vi "Main.vi"() -> ()   [LabVIEW 2016]
uses:
  <vilib>/picture/picture.llb/imagedata.ctl
panel:
  in  "Path 2":path
  in  "image data 2":T1 caption="图像数据"
  in  "Rectangle 2":T2
  out "Picture 2":picture
  in  "pConvertInfo In 4":T3
  in  "pConvertInfo In 3":T3
  out "frameHandle 2":i64
  out "Acquired Frames/s 2":dbl
  out "ResumeFlag 2":bool
  out "hDev 2":i64
  out "hIFDev 2":i64
  in  "ExposureAuto 2":i32(ring)
  in  "DeviceScanType 2":i32(ring) items=["Areascan", "Linescan"]
  out "InterfaceOpened 2":bool
  in  "Height 2":i32
  in  "Width 2":i32
  in  "PixelFormat 2":i32(ring)
  in  "GainRaw 2":dbl
  in  "ExposureTime 2":dbl
  out "IsGrabbing 2":bool
  out "TrigModeOn 2":bool
  in  "DeviceOpened 2":bool
  in  "DeviceList 2":i64(ring)
  out "ResumeFlag":bool
  in  "Path":path
  in  "SavePic":bool
  in  "pConvertInfo In 2":T3
  out "frameHandle":i64
  in  "DeviceInterfaceType":u16(ring) items=["GigE", "U3v", "CameraLink", "CXP"]
  in  "ExposureAuto":i32(ring)
  out "QuitFlag":bool
  in  "pConvertInfo In":T3
  in  "image data":T1 caption="图像数据"
  in  "Rectangle":T2
  in  "DeviceScanType":i32(ring) items=["Areascan", "Linescan"]
  out "InterfaceOpened":bool
  out "hDev":i64
  out "nInterfaceNum":u32
  out "hIFDev":i64
  out "interfaceKeyList":string[](array[string])
  out "HasInterface":bool
  out "Picture":picture
  out "Acquired Frames/s":dbl
  in  "TriggerSource":i32(ring)
  in  "ExecuteSoftTrig":bool
  in  "CloseTrig":bool
  in  "OpenTrig":bool
  in  "Stop":bool
  in  "Play":bool
  in  "Quit":bool
  in  "Height":i32
  in  "Width":i32
  in  "PixelFormat":i32(ring)
  in  "GainRaw":dbl
  in  "ExposureTime":dbl
  out "IsGrabbing":bool
  out "TrigModeOn":bool
  out "error out":errorcluster
  in  "error in":errorcluster
  in  "Close":bool
  in  "Open":bool
  out "HasDevices":bool
  in  "DeviceOpened":bool
  in  "DeviceList":i64(ring)
  in  "Discovery":bool
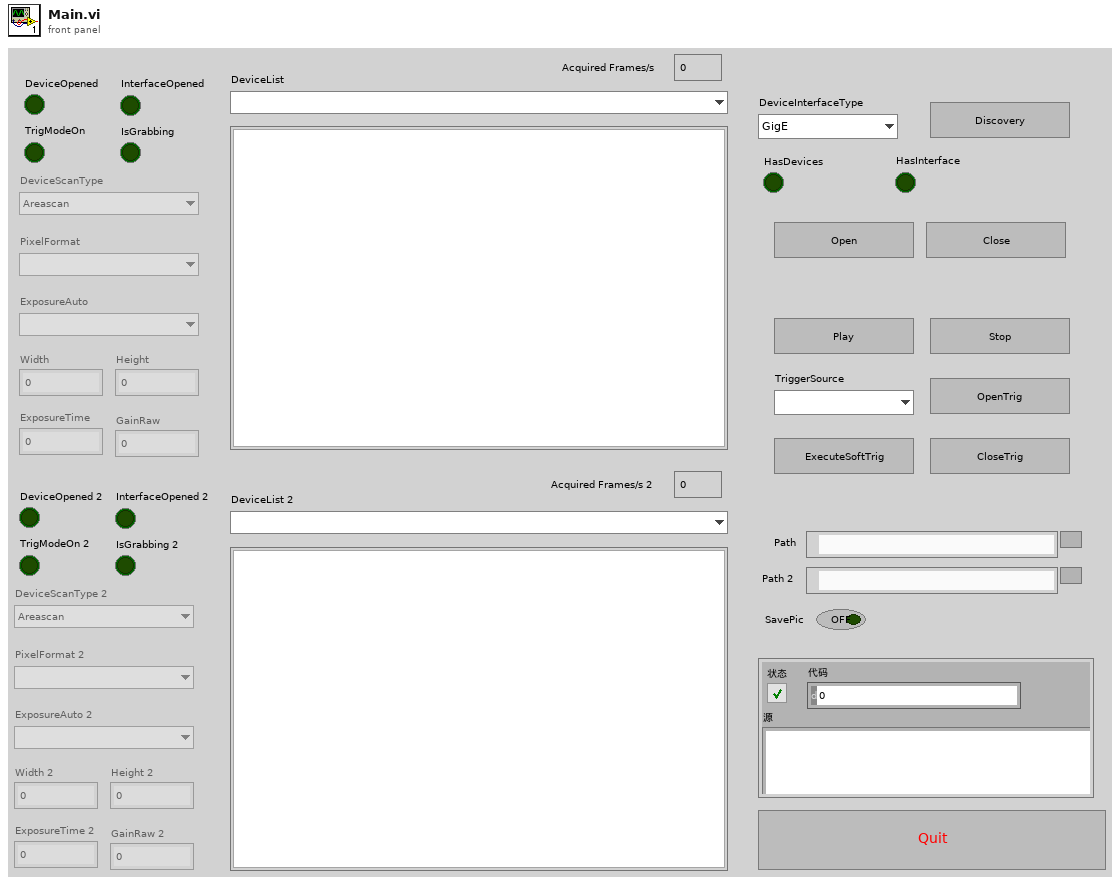
[diagram p1: front panel]
types:
  T1 = typedef "imagedata.ctl" = cluster{"image type":i32, "image depth":i32, "image":u8[], "mask":u8[], "colors":u32[], "Rectangle":cluster{"left":i16, "top":i16, "right":i16, "bottom":i16}}
  T2 = cluster{"left":i16, "top":i16, "right":i16, "bottom":i16}
  T3 = cluster{"nWidth":u32, "nHeight":u32, "enSrcPixelType":u32, "nSrcDataLen":u32, "nPaddingX":u32, "nPaddingY":u32, "eBayerDemosaic":u32, "eDstPixelFormat":u32, "nDstBufSize":u32, "nDstDataLen":u32, "nReserved0":u32, "nReserved1":u32, "nReserved2":u32, "nReserved3":u32, "nReserved4":u32, "nReserved5":u32, "nReserved6":u32, "nReserved7":u32}
  T4 = cluster{"blockId":u64, "status":u32, "width":u32, "height":u32, "size":u32, "pixelFormat":u32, "timeStamp":u64, "chunkCount":u32, "paddingX":u32, "paddingY":u32, "recvFrameTime":u32}
  T5 = cluster{"blockId":u64, "status":u32, "width":u32, "height":u32, "size":u32, "pixelFormat":i32, "timeStamp":u64, "chunkCount":u32, "paddingX":u32, "paddingY":u32, "recvFrameTime":u32}
  T6 = enum8{"Enabled", "Disabled", "Disabled and Grayed Out"}
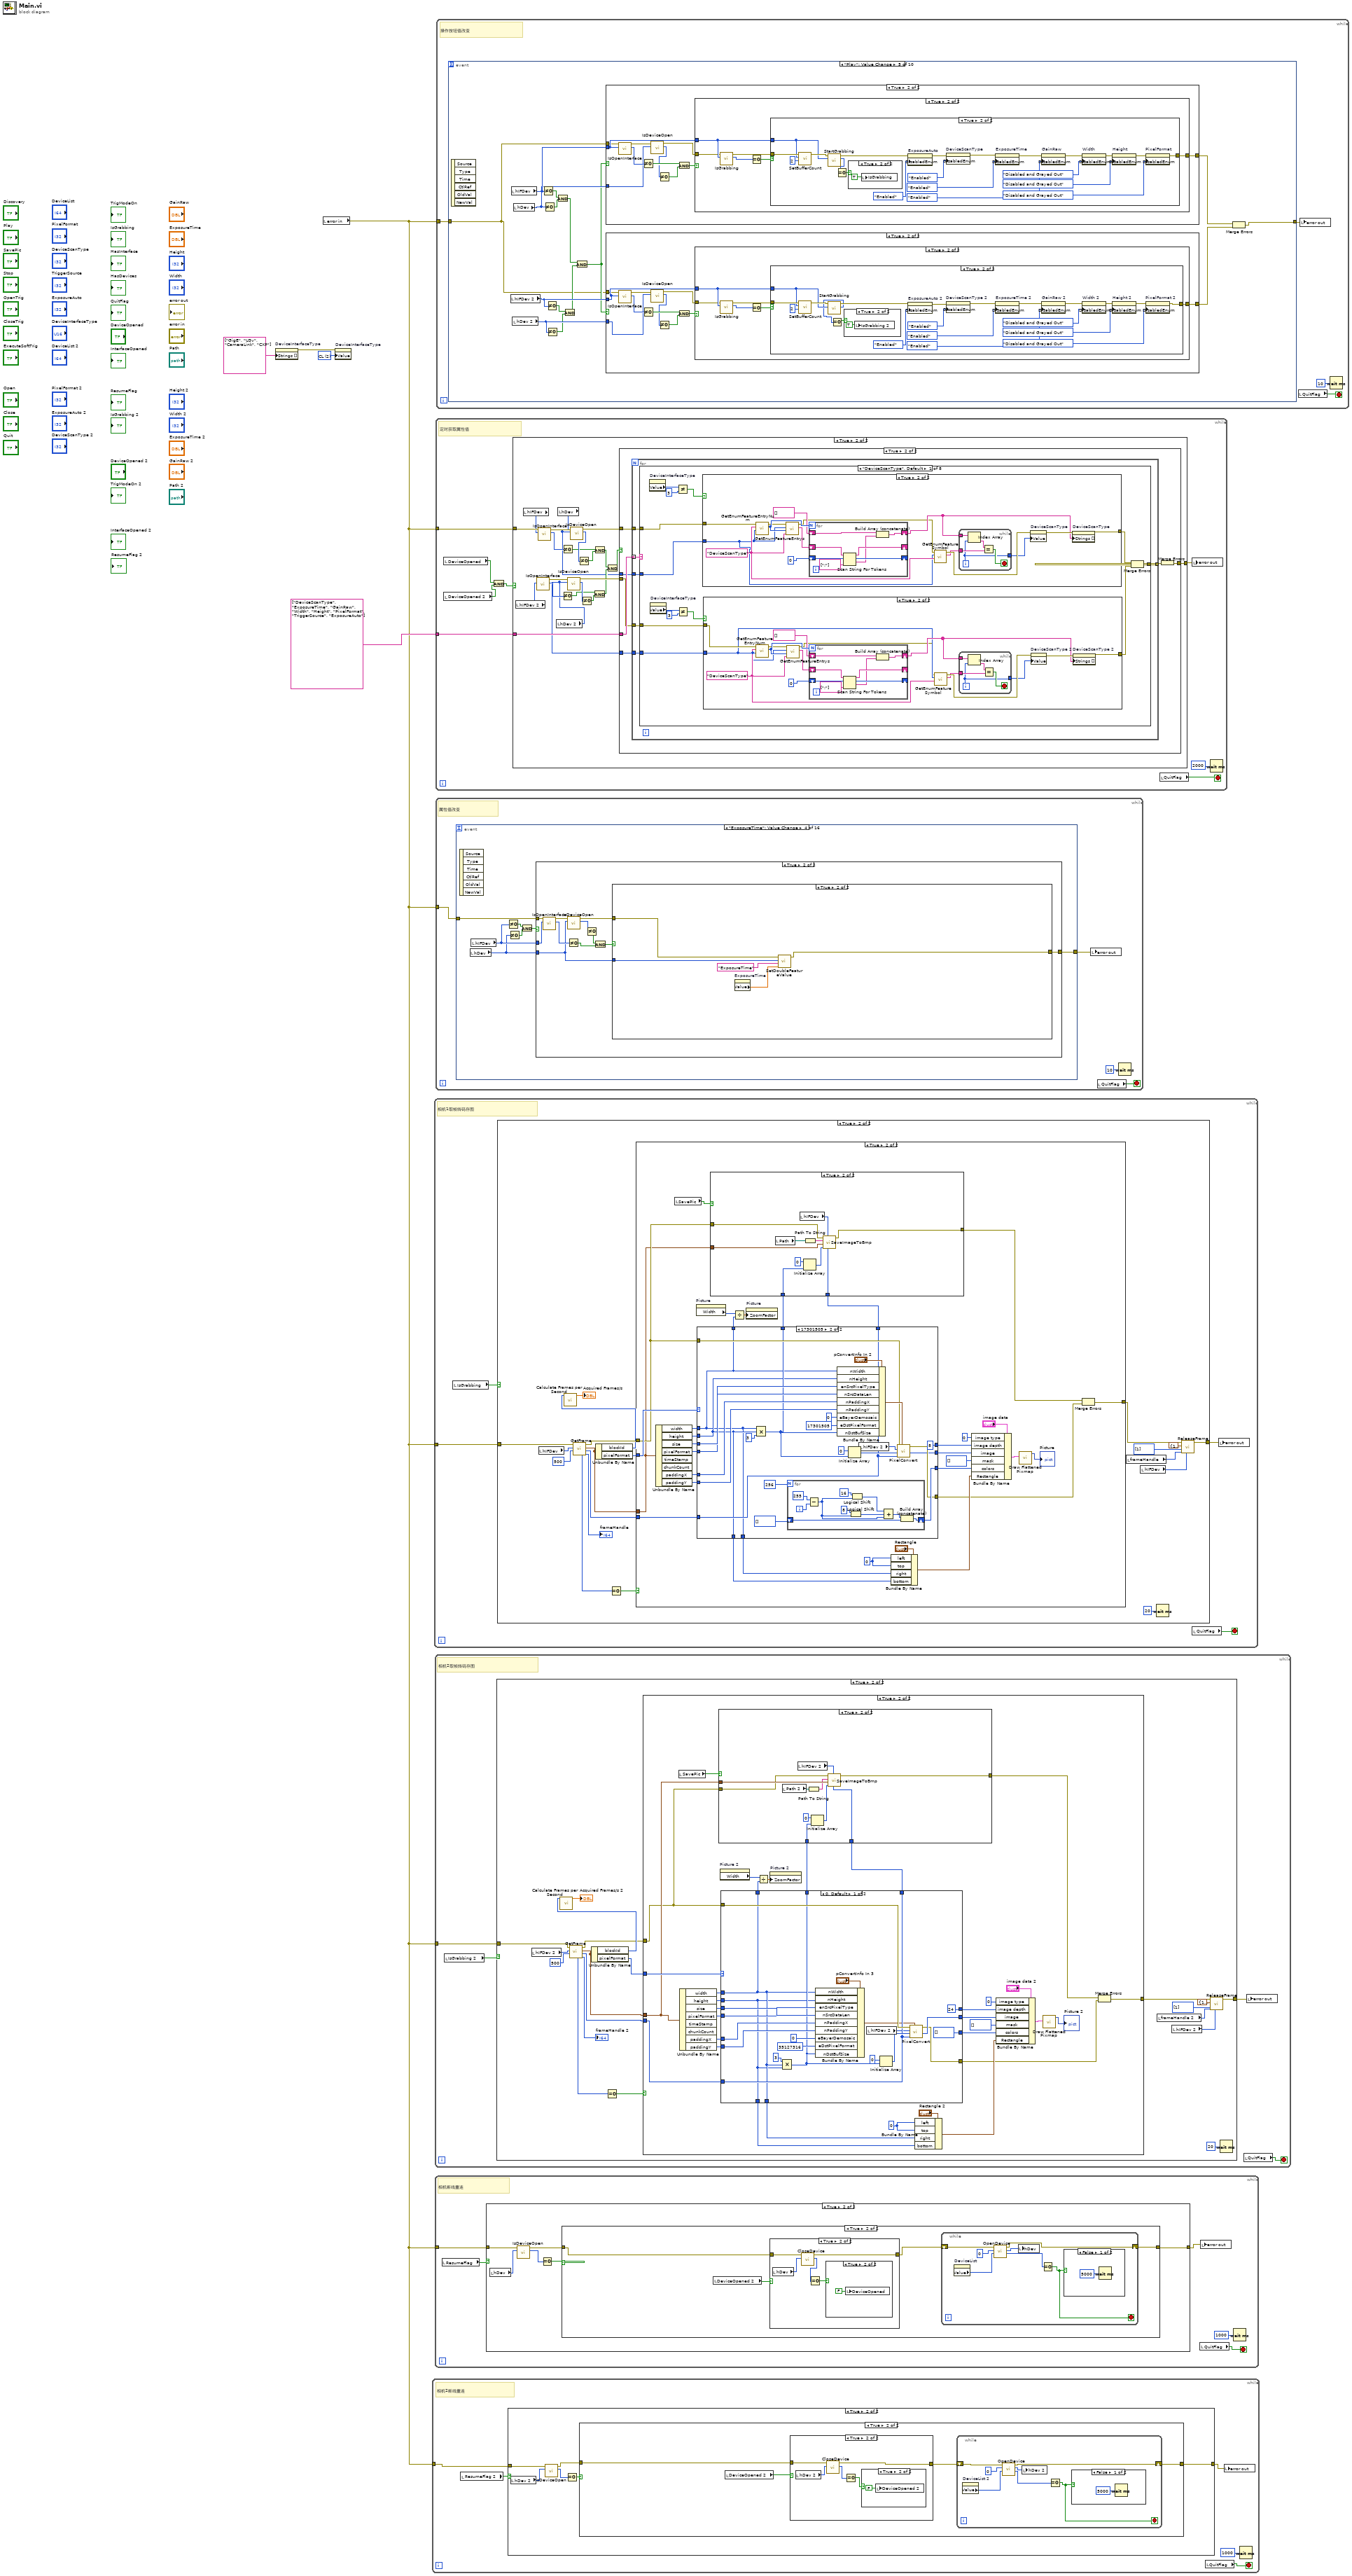
[diagram p0: block diagram]
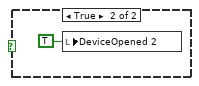
[diagram p4: hidden frame]
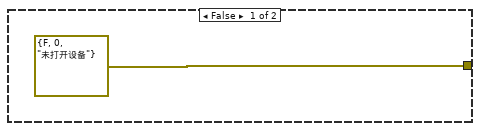
[diagram p7: hidden frame]
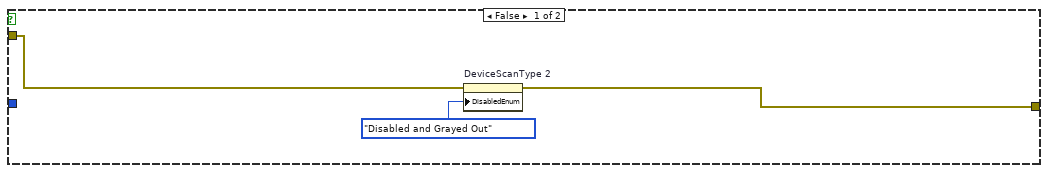
[diagram p9: hidden frame]
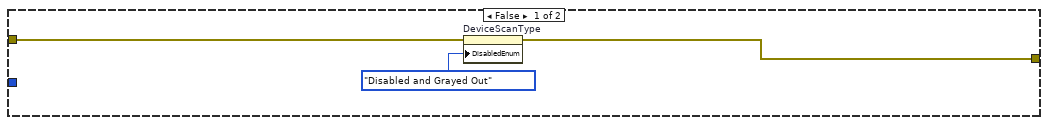
[diagram p10: hidden frame]
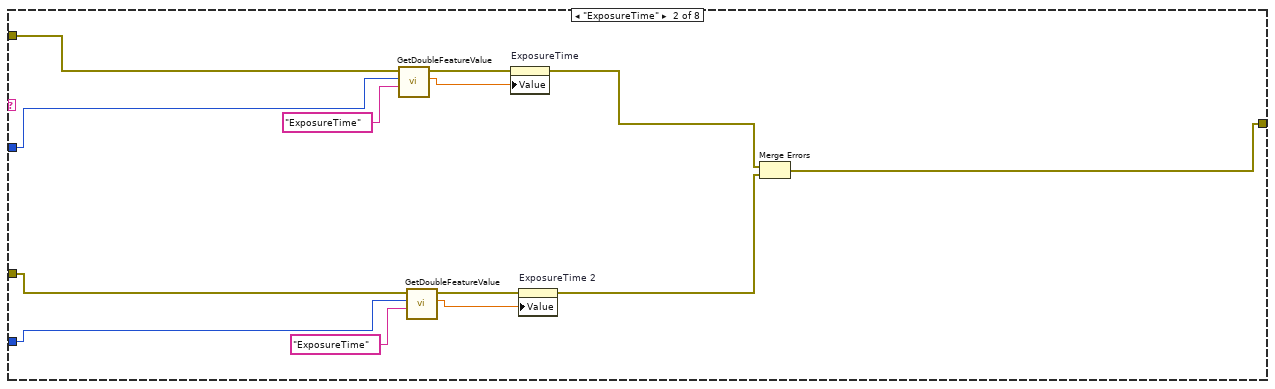
[diagram p11: hidden frame]
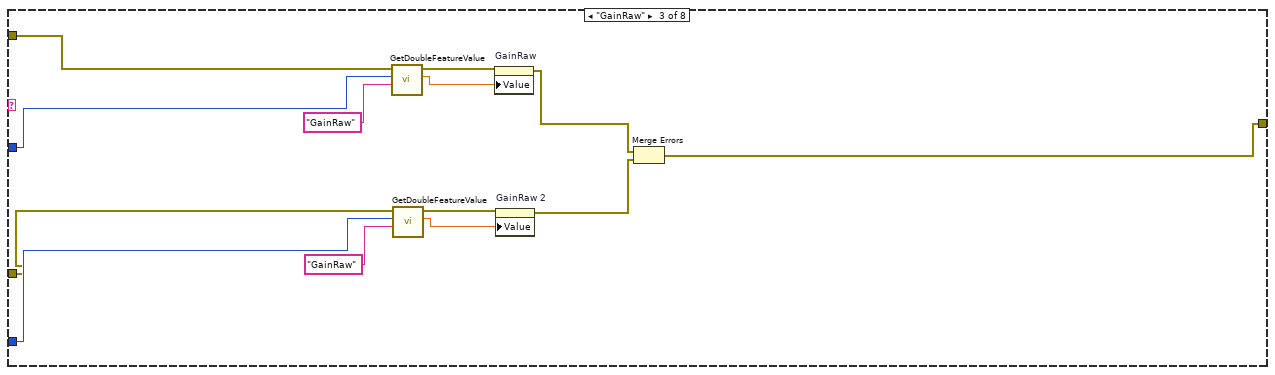
[diagram p12: hidden frame]
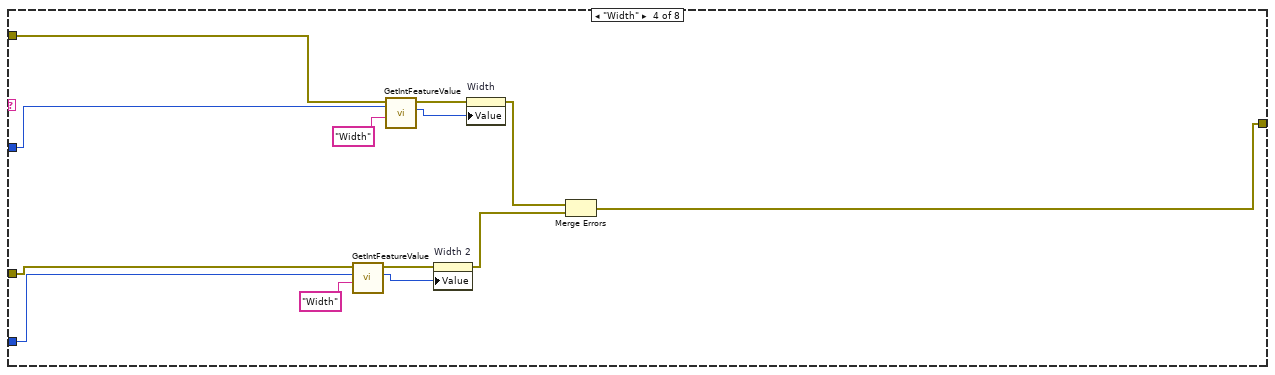
[diagram p13: hidden frame]
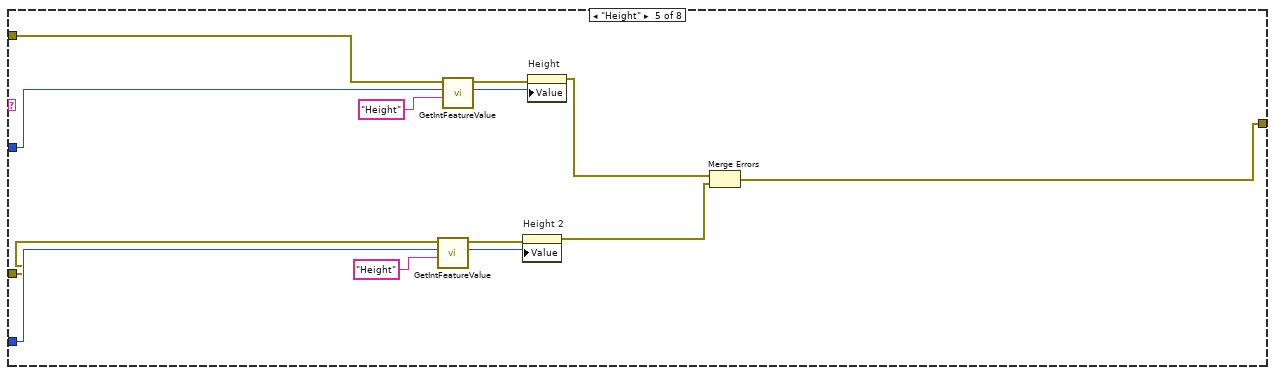
[diagram p14: hidden frame]
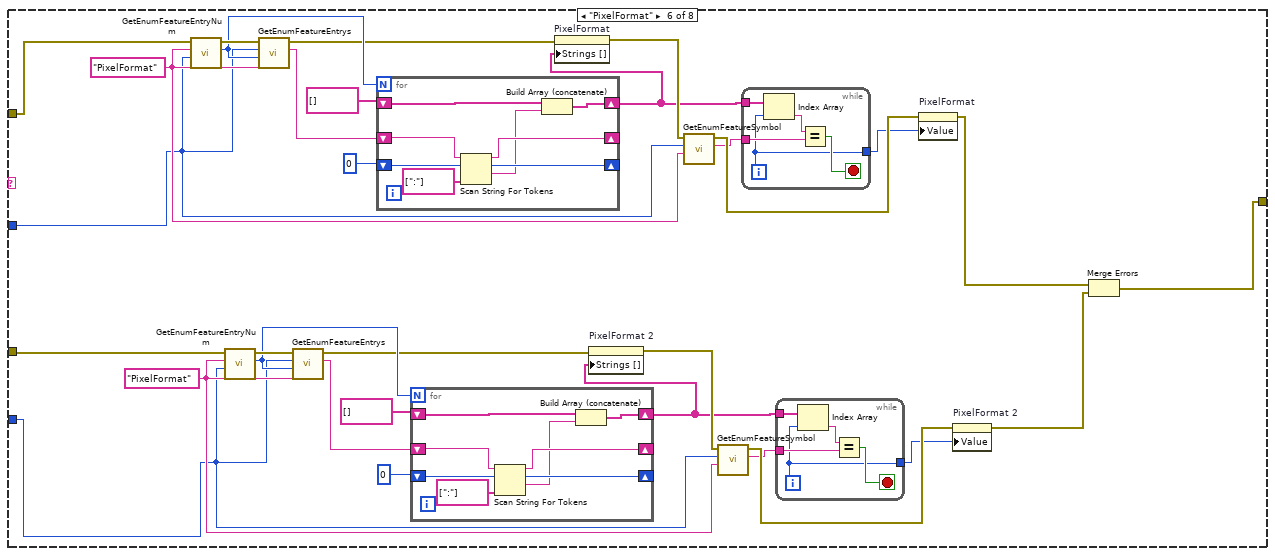
[diagram p15: hidden frame]
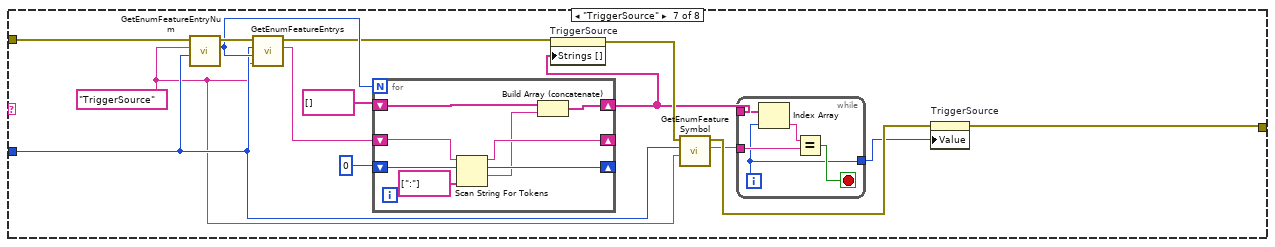
[diagram p16: hidden frame]
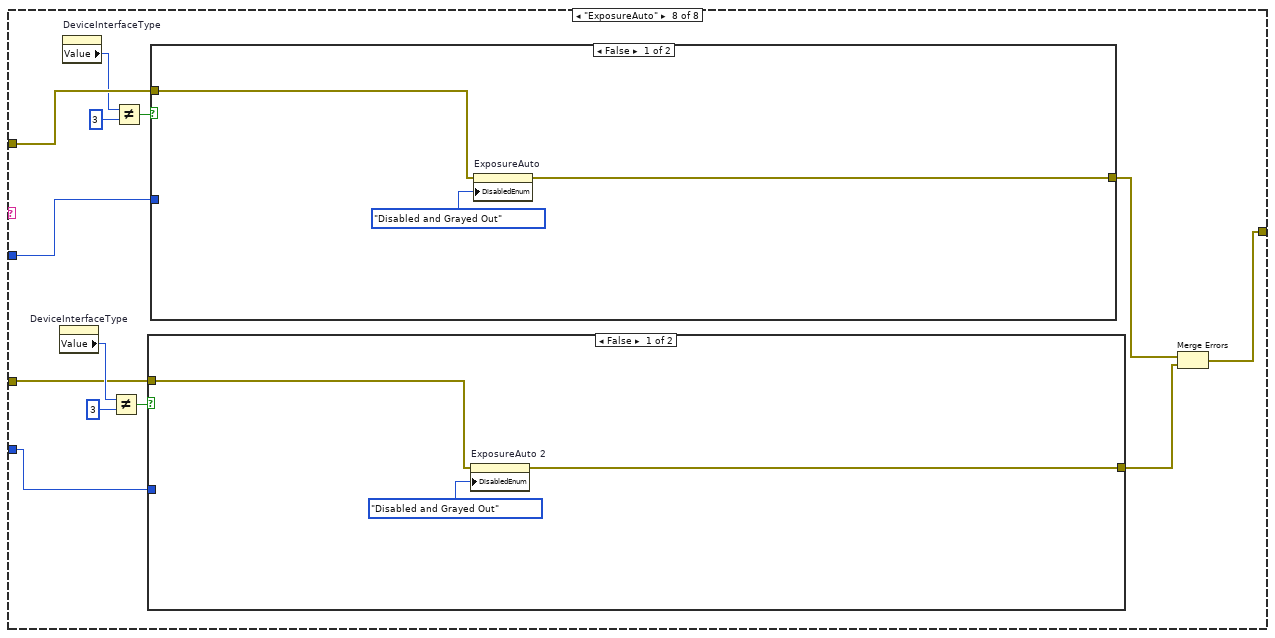
[diagram p17: hidden frame]
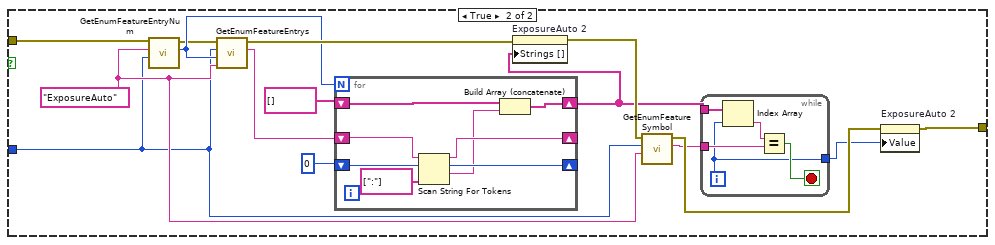
[diagram p18: hidden frame]
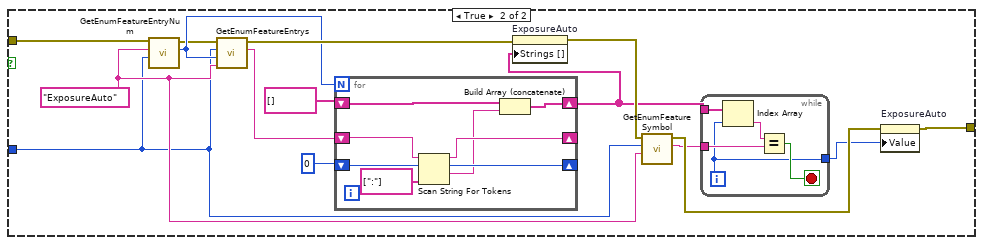
[diagram p19: hidden frame]
diagram:
  w3 = u16 2 items=["GigE", "U3v", "CL", "CXP"] ("DeviceInterfaceType")
  n1 = property on="DeviceInterfaceType" class="Ring (strict)"("Strings []"=string[] ["GigE", "U3v", "CameraLink", "CXP"]) -> (error out=w2:errorcluster)  [unwired: 2 in, 1 out]
  n2 = local read "error in"() -> (w1:errorcluster)
  n3 = property on="DeviceInterfaceType" class="Ring (strict)"(error in=w2, "Value"=w3) -> ()  [unwired: 1 in, 2 out]
  n4 = while {
    tunnel: w1 -> [w7]
    stop <- w10 stop-if-true
    # "相机2断线重连"
    n5 = local read "ResumeFlag 2"() -> (w8:bool)
    n6 = case shown="True" w8 {
      tunnel: [w11 w14] -> w6
      tunnel: w7 -> [w11 w13]
      frame False {
      }
      frame True {
        n7 = local read "hDev 2"() -> (w17:i64)
        n8 = call "IsDeviceOpen.vi"("dev handle"=w17, "error in (no error)"=w13) -> ("return type"=w16:i8, "error out"=w12:errorcluster)  [unwired: 8 in]
        n9 = Equal To 0?(x=w16) -> (x = 0?=w15:bool)
        n10 = case shown="True" w15 {
          tunnel: [w18 w20] -> w14
          tunnel: w12 -> [w18 w19]
          frame False {
          }
          frame True {
            n11 = local read "DeviceOpened 2"() -> (w21:bool)
            n12 = case shown="True" w21 {
              tunnel: [w32 w35] -> w22
              tunnel: w19 -> [w32 w33]
              frame False {
              }
              frame True {
                n13 = local read "hDev 2"() -> (w37:i64)
                n14 = call "CloseDevice.vi"("dev handle"=w37, "error in (no error)"=w33) -> ("return type"=w36:i32, "error out"=w35:errorcluster)  [unwired: 8 in]
                n15 = Equal To 0?(x=w36) -> (x = 0?=w34:bool)
                n16 = case shown="True" w34 {
                  frame False {
                  }
                  frame True {
                    n17 = local write "DeviceOpened 2"(FALSE ("DeviceOpened 2")) -> ()
                  }
                }
              }
            }
            n18 = while {
              shift-right: [w24] -> w20
              shift-left: w22 -> [w29]
              stop <- w23 stop-if-true
              n19 = property on="DeviceList 2" class="Ring (strict)"() -> ("Value"=w28:i64)  [unwired: 2 in, 2 out]
              n20 = call "OpenDevice.vi"("pIdentifier"=w28, "mode"=0, "error in (no error)"=w29) -> ("return type"=w25:i32, "hDev"=w26:i64, "error out"=w24:errorcluster)  [unwired: 6 in]
              n21 = local write "hDev 2"(w26) -> ()
              n22 = Equal To 0?(x=w25) -> (x = 0?=w23:bool)
              n23 = case shown="False" w23 {
                frame False {
                  n24 = Wait (ms)(milliseconds to wait=u32 5000 ("等待时间（毫秒）")) -> ()  [unwired: 1 out]
                }
                frame True {
                  n25 = local write "DeviceOpened 2"(TRUE ("DeviceOpened 2")) -> ()
                }
              }
            }
          }
        }
      }
    }
    n26 = local read "QuitFlag"() -> (w10:bool)
    n27 = local write "error out"(w6) -> ()
    n28 = Wait (ms)(milliseconds to wait=u32 1000 ("等待时间（毫秒）")) -> ()  [unwired: 1 out]
  }
  n29 = while {
    tunnel: w1 -> [w42]
    stop <- w40 stop-if-true
    # "相机1取帧转码存图"
    n30 = local read "IsGrabbing"() -> (w39:bool)
    n31 = case shown="True" w39 {
      tunnel: w42 -> [w43 w49]
      tunnel: [w43 w52] -> w41
      frame False {
      }
      frame True {
        n32 = local read "hIFDev"() -> (w47:i64)
        n33 = call "GetFrame.vi"("timeoutMS"=u32 500, "handle"=w47, "error in (no error)"=w49) -> ("frameHandle"=→"frameHandle":i64, "pData"=w59:u8[], "pLbFrame out"=w60:T5, "error out"=w54:errorcluster, "return type"=w62:i32)  [unwired: 4 in]
        n34 = Unbundle By Name(w60) -> ("blockId"=w51:u64, "pixelFormat"=w55:i32)
        n35 = call <vilib>:"Calculate Frames per Second.vi"("Buffer Number"=w51) -> ("Acquired Frames/s"=→"Acquired Frames/s":dbl)  [unwired: 8 in, 2 out]
        n36 = Equal To 0?(x=w62) -> (x = 0?=w61:bool)
        n37 = case shown="True" w61 {
          tunnel: w60 -> [_ w76]
          tunnel: w59 -> [_ w79]
          tunnel: w55 -> [_ w94]
          tunnel: w54 -> [w64 w83]
          tunnel: [w64 w80] -> w53
          frame False {
            n38 = Wait (ms)(milliseconds to wait=u32 2000 ("等待时间（毫秒）")) -> ()  [unwired: 1 out]
          }
          frame True {
            w92 = i16 0 ("left")
            n39 = Unbundle By Name(w76) -> ("width"=w75:u32, "height"=w74:u32, "size"=w73:u32, "pixelFormat"=w72:i32, "paddingX"=w71:u32, "paddingY"=w70:u32)  [unwired: 2 out]
            n40 = local read "SavePic"() -> (w78:bool)
            n41 = property on="Picture" class="Pict"() -> ("Width"=w67:u32)  [unwired: 2 in, 2 out]
            n42 = case shown="17301505" w94 {
              tunnel: [i32[] [] w149] -> w87
              tunnel: w79 -> [w118 w139]
              tunnel: [w123 w140] -> w84
              tunnel: [24 8] -> w85
              tunnel: w83 -> [w120 w142]
              tunnel: [w119 w141] -> w81
              tunnel: [w118 w139] -> w77
              tunnel: w75 -> [w110 w130]
              tunnel: w74 -> [w109 w131]
              tunnel: w73 -> [w116 w137]
              tunnel: w72 -> [w115 w136]
              tunnel: w71 -> [w114 w135]
              tunnel: w70 -> [w113 w134]
              tunnel: [w110 w130] -> w69
              tunnel: [w109 w131] -> w68
              tunnel: [w110 w130] -> w66
              tunnel: [w111 w133] -> w65
              frame 0, Default {
                n43 = Compound Arithmetic op=MULTIPLY(u32 3 ("value"), w110, w109) -> (w111:u32)
                n44 = Bundle By Name(cluster="pConvertInfo In", "nWidth"=w110, "nHeight"=w109, "enSrcPixelType"=w115, "nSrcDataLen"=w116, "nPaddingX"=w114, "nPaddingY"=w113, "eBayerDemosaic"=u32 0, "eDstPixelFormat"=u32 35127316 ("enDstPixelType"), "nDstBufSize"=w111) -> (w117:T3)
                n45 = local read "hIFDev 2"() -> (w108:i64)
                n46 = Initialize Array(u8 0, w111) -> (w124:u8[])
                n47 = call "PixelConvert.vi"("lbPstPixelConvertParam"=w117, "pSrcData"=w118, "pDstBuf"=w124, "Interface handle"=w108, "error in (no error)"=w120) -> ("pDstBuf out"=w123:u8[], "error out"=w119:errorcluster)  [unwired: 5 in]
              }
              frame 17301505 {
                n48 = Compound Arithmetic op=MULTIPLY(w130, w131, u32 3 ("value")) -> (w133:u32)
                n49 = for {
                  N: 256 -> [_]
                  shift-right: [w156] -> w149
                  shift-left: i32[] [] ("数组") -> [w155]
                  i -> [w152]
                  n50 = Subtract(x=255, y=w152) -> (x-y=w153:i32)
                  n51 = Logical Shift(y=i16 8, x=w153) -> (x << y=w158:i32)
                  n52 = Logical Shift(y=16 ("x"), x=w153) -> (x << y=w159:i32)
                  n53 = Compound Arithmetic op=ADD(w159, w158, w153) -> (w157:i32)
                  n54 = Build Array (concatenate)(w157, w155) -> (w156:i32[])
                }
                n55 = Bundle By Name(cluster="pConvertInfo In 2", "nWidth"=w130, "nHeight"=w131, "enSrcPixelType"=w136, "nSrcDataLen"=w137, "nPaddingX"=w135, "nPaddingY"=w134, "eBayerDemosaic"=u32 0, "eDstPixelFormat"=u32 17301505 ("enDstPixelType"), "nDstBufSize"=w133) -> (w143:T3)
                n56 = Initialize Array(u8 0, w133) -> (w144:u8[])
                n57 = local read "hIFDev 2"() -> (w129:i64)
                n58 = call "PixelConvert.vi"("lbPstPixelConvertParam"=w143, "pSrcData"=w139, "pDstBuf"=w144, "Interface handle"=w129, "error in (no error)"=w142) -> ("pDstBuf out"=w140:u8[], "error out"=w141:errorcluster)  [unwired: 5 in]
              }
            }
            n59 = case shown="True" w78 {
              tunnel: w83 -> [w97 w107]
              tunnel: [w97 w106] -> w82
              tunnel: w76 -> [_ w105]
              tunnel: w77 -> [_ w104]
              tunnel: w65 -> [_ w98]
              frame False {
              }
              frame True {
                n60 = local read "Path"() -> (w103:path)
                n61 = local read "hIFDev"() -> (w101:i64)
                n62 = Initialize Array(u8 0, w98) -> (w99:u8[])
                n63 = Path To String(path=w103) -> (string=w102:string)
                n64 = call "SaveImageToBmp.vi"("pSrcData"=w104, "interface handle"=w101, "pDstBuf"=w99, "pLbFrame"=w105, "filePath"=w102, "error in (no error)"=w107) -> ("error out"=w106:errorcluster)  [unwired: 4 in, 1 out]
              }
            }
            n65 = Divide(x=w67, y=w66) -> (x/y=w95:dbl)
            n66 = property on="Picture" class="Pict"("ZoomFactor"=w95) -> ()  [unwired: 2 in, 2 out]
            n67 = Bundle By Name(cluster="Rectangle", "left"=w92, "top"=w92, "right"=w69, "bottom"=w68) -> (w88:T2)
            n68 = Bundle By Name(cluster="image data", "image type"=0, "image depth"=w85, "image"=w84, "mask"=u8[] [], "colors"=w87, "Rectangle"=w88) -> (w90:T1)
            n69 = call <vilib>:"Draw Flattened Pixmap.vi"("image data"=w90) -> ("new picture"=→"Picture":picture)  [unwired: 8 in]
            n70 = Merge Errors(w82, w81) -> (w80:errorcluster)
          }
        }
        n71 = local read "frameHandle"() -> (w48:i64)
        n72 = local read "hIFDev"() -> (w57:i64)
        n73 = Wait (ms)(milliseconds to wait=u32 20 ("等待时间（毫秒）")) -> ()  [unwired: 1 out]
        n74 = call "ReleaseFrame.vi"("interface handle"=w57, "frameHandle"=w48, "pData"=u8[] [1], "pLbFrame"=T4 {"blockId"=1, "status"=0, "width"=0, "height"=0, "size"=0, "pixelFormat"=0, "timeStamp"=0, "chunkCount"=0, "paddingX"=0, "paddingY"=0, "recvFrameTime"=0}, "error in (no error)"=w53) -> ("error out"=w52:errorcluster)  [unwired: 6 in]
      }
    }
    n75 = local read "QuitFlag"() -> (w40:bool)
    n76 = local write "error out"(w41) -> ()
  }
  n77 = while {
    tunnel: w1 -> [w164]
    stop <- w162 stop-if-true
    # "相机2取帧转码存图"
    n78 = local read "IsGrabbing 2"() -> (w165:bool)
    n79 = case shown="True" w165 {
      tunnel: w164 -> [w166 w178]
      tunnel: [w166 w167] -> w163
      frame False {
      }
      frame True {
        n80 = local read "hIFDev 2"() -> (w181:i64)
        n81 = call "GetFrame.vi"("timeoutMS"=u32 500, "handle"=w181, "error in (no error)"=w178) -> ("frameHandle"=→"frameHandle 2":i64, "pData"=w177:u8[], "pLbFrame out"=w176:T5, "error out"=w175:errorcluster, "return type"=w185:i32)  [unwired: 4 in]
        n82 = Unbundle By Name(w176) -> ("blockId"=w179:u64, "pixelFormat"=w174:i32)
        n83 = call <vilib>:"Calculate Frames per Second.vi"("Buffer Number"=w179) -> ("Acquired Frames/s"=→"Acquired Frames/s 2":dbl)  [unwired: 8 in, 2 out]
        n84 = Equal To 0?(x=w185) -> (x = 0?=w182:bool)
        n85 = case shown="True" w182 {
          tunnel: w177 -> [_ w196]
          tunnel: w176 -> [_ w192]
          tunnel: w175 -> [w186 w191]
          tunnel: w174 -> [_ w195]
          tunnel: [w186 w187] -> w172
          frame False {
          }
          frame True {
            w215 = i16 0 ("left")
            n86 = local read "SavePic"() -> (w194:bool)
            n87 = Unbundle By Name(w192) -> ("width"=w206:u32, "height"=w205:u32, "size"=w204:u32, "pixelFormat"=w203:i32, "paddingX"=w202:u32, "paddingY"=w201:u32)  [unwired: 2 out]
            n88 = property on="Picture 2" class="Pict"() -> ("Width"=w198:u32)  [unwired: 2 in, 2 out]
            n89 = case shown="0, Default" w195 {
              tunnel: [i32[] [] w271] -> w210
              tunnel: w196 -> [w240 w261]
              tunnel: [w245 w262] -> w207
              tunnel: [24 8] -> w208
              tunnel: w191 -> [w242 w264]
              tunnel: [w241 w263] -> w188
              tunnel: [w240 w261] -> w190
              tunnel: w206 -> [w232 w252]
              tunnel: w205 -> [w231 w253]
              tunnel: w204 -> [w238 w259]
              tunnel: w203 -> [w237 w258]
              tunnel: w202 -> [w236 w257]
              tunnel: w201 -> [w235 w256]
              tunnel: [w232 w252] -> w200
              tunnel: [w231 w253] -> w199
              tunnel: [w232 w252] -> w197
              tunnel: [w233 w255] -> w193
              frame 0, Default {
                n90 = Compound Arithmetic op=MULTIPLY(u32 3 ("value"), w232, w231) -> (w233:u32)
                n91 = Bundle By Name(cluster="pConvertInfo In 3", "nWidth"=w232, "nHeight"=w231, "enSrcPixelType"=w237, "nSrcDataLen"=w238, "nPaddingX"=w236, "nPaddingY"=w235, "eBayerDemosaic"=u32 0, "eDstPixelFormat"=u32 35127316 ("enDstPixelType"), "nDstBufSize"=w233) -> (w239:T3)
                n92 = local read "hIFDev 2"() -> (w230:i64)
                n93 = Initialize Array(u8 0, w233) -> (w246:u8[])
                n94 = call "PixelConvert.vi"("lbPstPixelConvertParam"=w239, "pSrcData"=w240, "pDstBuf"=w246, "Interface handle"=w230, "error in (no error)"=w242) -> ("pDstBuf out"=w245:u8[], "error out"=w241:errorcluster)  [unwired: 5 in]
              }
              frame 17301505 {
                n95 = Compound Arithmetic op=MULTIPLY(w252, w253, u32 3 ("value")) -> (w255:u32)
                n96 = for {
                  N: 256 -> [_]
                  shift-right: [w278] -> w271
                  shift-left: i32[] [] ("数组") -> [w277]
                  i -> [w274]
                  n97 = Subtract(x=255, y=w274) -> (x-y=w275:i32)
                  n98 = Logical Shift(y=i16 8, x=w275) -> (x << y=w280:i32)
                  n99 = Logical Shift(y=16 ("x"), x=w275) -> (x << y=w281:i32)
                  n100 = Compound Arithmetic op=ADD(w281, w280, w275) -> (w279:i32)
                  n101 = Build Array (concatenate)(w279, w277) -> (w278:i32[])
                }
                n102 = Bundle By Name(cluster="pConvertInfo In 4", "nWidth"=w252, "nHeight"=w253, "enSrcPixelType"=w258, "nSrcDataLen"=w259, "nPaddingX"=w257, "nPaddingY"=w256, "eBayerDemosaic"=u32 0, "eDstPixelFormat"=u32 17301505 ("enDstPixelType"), "nDstBufSize"=w255) -> (w265:T3)
                n103 = Initialize Array(u8 0, w255) -> (w266:u8[])
                n104 = local read "hIFDev 2"() -> (w251:i64)
                n105 = call "PixelConvert.vi"("lbPstPixelConvertParam"=w265, "pSrcData"=w261, "pDstBuf"=w266, "Interface handle"=w251, "error in (no error)"=w264) -> ("pDstBuf out"=w262:u8[], "error out"=w263:errorcluster)  [unwired: 5 in]
              }
            }
            n106 = case shown="True" w194 {
              tunnel: w193 -> [_ w228]
              tunnel: w192 -> [_ w227]
              tunnel: w191 -> [w219 w226]
              tunnel: w190 -> [_ w222]
              tunnel: [w219 w220] -> w189
              frame False {
              }
              frame True {
                n107 = local read "Path 2"() -> (w225:path)
                n108 = local read "hIFDev 2"() -> (w221:i64)
                n109 = Path To String(path=w225) -> (string=w224:string)
                n110 = Initialize Array(u8 0, w228) -> (w223:u8[])
                n111 = call "SaveImageToBmp.vi"("pSrcData"=w222, "interface handle"=w221, "pDstBuf"=w223, "pLbFrame"=w227, "filePath"=w224, "error in (no error)"=w226) -> ("error out"=w220:errorcluster)  [unwired: 4 in, 1 out]
              }
            }
            n112 = Divide(x=w198, y=w197) -> (x/y=w217:dbl)
            n113 = property on="Picture 2" class="Pict"("ZoomFactor"=w217) -> ()  [unwired: 2 in, 2 out]
            n114 = Bundle By Name(cluster="Rectangle 2", "left"=w215, "top"=w215, "right"=w200, "bottom"=w199) -> (w211:T2)
            n115 = Bundle By Name(cluster="image data 2", "image type"=0, "image depth"=w208, "image"=w207, "mask"=u8[] [], "colors"=w210, "Rectangle"=w211) -> (w213:T1)
            n116 = call <vilib>:"Draw Flattened Pixmap.vi"("image data"=w213) -> ("new picture"=→"Picture 2":picture)  [unwired: 8 in]
            n117 = Merge Errors(w189, w188) -> (w187:errorcluster)
          }
        }
        n118 = local read "frameHandle 2"() -> (w170:i64)
        n119 = local read "hIFDev 2"() -> (w169:i64)
        n120 = call "ReleaseFrame.vi"("interface handle"=w169, "frameHandle"=w170, "pData"=u8[] [1], "pLbFrame"=T4 {"blockId"=1, "status"=0, "width"=0, "height"=0, "size"=0, "pixelFormat"=0, "timeStamp"=0, "chunkCount"=0, "paddingX"=0, "paddingY"=0, "recvFrameTime"=0}, "error in (no error)"=w172) -> ("error out"=w167:errorcluster)  [unwired: 6 in]
        n121 = Wait (ms)(milliseconds to wait=u32 20 ("等待时间（毫秒）")) -> ()  [unwired: 1 out]
      }
    }
    n122 = local read "QuitFlag"() -> (w162:bool)
    n123 = local write "error out"(w163) -> ()
  }
  n124 = while {
    tunnel: w1 -> [w285]
    stop <- w288 stop-if-true
    # "相机断线重连"
    n125 = local read "ResumeFlag"() -> (w286:bool)
    n126 = case shown="True" w286 {
      tunnel: w285 -> [w289 w292]
      tunnel: [w289 w290] -> w284
      frame False {
      }
      frame True {
        n127 = local read "hDev"() -> (w295:i64)
        n128 = call "IsDeviceOpen.vi"("dev handle"=w295, "error in (no error)"=w292) -> ("return type"=w294:i8, "error out"=w291:errorcluster)  [unwired: 8 in]
        n129 = Equal To 0?(x=w294) -> (x = 0?=w293:bool)
        n130 = case shown="True" w293 {
          tunnel: w291 -> [w296 w297]
          tunnel: [w296 w298] -> w290
          frame False {
          }
          frame True {
            n131 = local read "DeviceOpened 2"() -> (w300:bool)
            n132 = case shown="True" w300 {
              tunnel: [w310 w312] -> w299
              tunnel: w297 -> [w310 w311]
              frame False {
              }
              frame True {
                n133 = local read "hDev"() -> (w315:i64)
                n134 = call "CloseDevice.vi"("dev handle"=w315, "error in (no error)"=w311) -> ("return type"=w313:i32, "error out"=w312:errorcluster)  [unwired: 8 in]
                n135 = Equal To 0?(x=w313) -> (x = 0?=w314:bool)
                n136 = case shown="True" w314 {
                  frame False {
                  }
                  frame True {
                    n137 = local write "DeviceOpened"(FALSE ("DeviceOpened")) -> ()
                  }
                }
              }
            }
            n138 = while {
              shift-right: [w302] -> w298
              shift-left: w299 -> [w303]
              stop <- w301 stop-if-true
              n139 = property on="DeviceList" class="Ring (strict)"() -> ("Value"=w305:i64)  [unwired: 2 in, 2 out]
              n140 = call "OpenDevice.vi"("pIdentifier"=w305, "mode"=0, "error in (no error)"=w303) -> ("return type"=w306:i32, "hDev"=w307:i64, "error out"=w302:errorcluster)  [unwired: 6 in]
              n141 = local write "hDev"(w307) -> ()
              n142 = Equal To 0?(x=w306) -> (x = 0?=w301:bool)
              n143 = case shown="False" w301 {
                frame False {
                  n144 = Wait (ms)(milliseconds to wait=u32 5000 ("等待时间（毫秒）")) -> ()  [unwired: 1 out]
                }
                frame True {
                  n145 = local write "DeviceOpened"(TRUE ("DeviceOpened")) -> ()
                }
              }
            }
          }
        }
      }
    }
    n146 = local read "QuitFlag"() -> (w288:bool)
    n147 = local write "error out"(w284) -> ()
    n148 = Wait (ms)(milliseconds to wait=u32 1000 ("等待时间（毫秒）")) -> ()  [unwired: 1 out]
  }
  n149 = while {
    tunnel: string[] ["DeviceScanType", "ExposureTime", "GainRaw", "Width", "Height", "PixelFormat", "TriggerSource", "ExposureAuto"] -> [w324]
    tunnel: w1 -> [w322]
    stop <- w321 stop-if-true
    # "定时获取属性值"
    n150 = local read "DeviceOpened"() -> (w318:bool)
    n151 = local read "DeviceOpened 2"() -> (w317:bool)
    n152 = And(x=w318, y=w317) -> (x .and. y?=w319:bool)
    n153 = case shown="True" w319 {
      tunnel: w324 -> [_ w347]
      tunnel: w322 -> [_ w345]
      tunnel: [errorcluster {"status"=FALSE, "code"=0, "source"="未打开设备"} ("错误常量") w346] -> w323
      frame False {
      }
      frame True {
        n154 = local read "hIFDev 2"() -> (w327:i64)
        n155 = local read "hIFDev"() -> (w329:i64)
        n156 = call "IsOpenInterface.vi"("interface handle"=w327) -> ("return type"=w336:i8, "error out"=w338:errorcluster)  [unwired: 9 in]
        n157 = call "IsOpenInterface.vi"("interface handle"=w329, "error in (no error)"=w345) -> ("return type"=w342:i8, "error out"=w344:errorcluster)  [unwired: 8 in]
        n158 = local read "hDev 2"() -> (w326:i64)
        n159 = local read "hDev"() -> (w328:i64)
        n160 = Not Equal To 0?(x=w336) -> (x != 0?=w334:bool)
        n161 = Not Equal To 0?(x=w342) -> (x != 0?=w340:bool)
        n162 = call "IsDeviceOpen.vi"("dev handle"=w326, "error in (no error)"=w338) -> ("return type"=w335:i8, "error out"=w337:errorcluster)  [unwired: 8 in]
        n163 = call "IsDeviceOpen.vi"("dev handle"=w328, "error in (no error)"=w344) -> ("return type"=w341:i8, "error out"=w343:errorcluster)  [unwired: 8 in]
        n164 = Not Equal To 0?(x=w341) -> (x != 0?=w339:bool)
        n165 = Not Equal To 0?(x=w335) -> (x != 0?=w333:bool)
        n166 = And(x=w334, y=w333) -> (x .and. y?=w331:bool)
        n167 = And(x=w340, y=w339) -> (x .and. y?=w332:bool)
        n168 = And(x=w332, y=w331) -> (x .and. y?=w330:bool)
        n169 = case shown="True" w330 {
          tunnel: w347 -> [_ w355]
          tunnel: [w348 w353] -> w346
          tunnel: w343 -> [w348 w352]
          tunnel: w328 -> [_ w351]
          tunnel: w337 -> [_ w349]
          tunnel: w326 -> [_ w350]
          frame False {
          }
          frame True {
            n170 = for {
              tunnel: w355 -> [w361] mode=indexing
              tunnel: [w360] -> w354 mode=indexing
              tunnel: w352 -> [w359]
              tunnel: w351 -> [w358]
              tunnel: w350 -> [w357]
              tunnel: w349 -> [w356]
              n171 = case shown="\"DeviceScanType\", Default" w361 {
                tunnel: [w362 w437 w450 w463 w476 w489 w549 w574] -> w360
                tunnel: w359 -> [w374 w446 w459 w472 w485 w506 w553 w586]
                tunnel: w358 -> [w373 w445 w458 w471 w484 w507 w552 w585]
                tunnel: w357 -> [w366 w441 w454 w466 w480 w492 _ w577]
                tunnel: w356 -> [w365 w440 w453 w467 w479 w493 _ w578]
                frame "DeviceScanType", Default {
                  n172 = property on="DeviceInterfaceType" class="Ring (strict)"() -> ("Value"=w371:u16)  [unwired: 2 in, 2 out]
                  n173 = property on="DeviceInterfaceType" class="Ring (strict)"() -> ("Value"=w368:u16)  [unwired: 2 in, 2 out]
                  n174 = Not Equal?(x=w371, y=3) -> (x != y?=w372:bool)
                  n175 = Not Equal?(x=w368, y=3) -> (x != y?=w369:bool)
                  n176 = case shown="True" w372 {
                    tunnel: w374 -> [w406 w418]
                    tunnel: w373 -> [_ w410]
                    tunnel: [w407 w414] -> w364
                    frame False {
                      n177 = property on="DeviceScanType" class="Ring (strict)"(error in=w406, "DisabledEnum"=T6."Disabled and Grayed Out" ("Disabled")) -> (error out=w407:errorcluster)  [unwired: 1 in, 1 out]
                    }
                    frame True {
                      w416 = "DeviceScanType" ("pFeatureName")
                      n178 = call "GetEnumFeatureEntryNum.vi"("handle"=w410, "pFeatureName"=w416, "error in (no error)"=w418) -> ("pEntryNum"=w421:u32, "error out"=w420:errorcluster)  [unwired: 7 in]
                      n179 = call "GetEnumFeatureEntrys.vi"("pFeatureName"=w416, "EntryNum"=w421, "handle"=w410, "error in (no error)"=w420) -> ("pLbEnumEntryList"=w422:string, "error out"=w409:errorcluster)  [unwired: 6 in]
                      n180 = for {
                        N: w421 -> [_]
                        shift-right: [w434] -> _
                        shift-left: 0 ("offset past token") -> [w435]
                        shift-right: [w432] -> _
                        shift-left: w422 -> [w433]
                        shift-right: [w430] -> w413
                        shift-left: string[] [] -> [w431]
                        n181 = Scan String For Tokens(6:string[] [":"] ("delimiters (\\s,\\t,\\r,\\n)"), 8:w435, 9:w433) -> (1:w429:string, 2:w434:i32, 3:w432:string)  [unwired: 3 in, 1 out]
                        n182 = Build Array (concatenate)(w431, w429) -> (w430:string[])
                      }
                      n183 = call "GetEnumFeatureSymbol.vi"("pFeatureName"=w416, "handle"=w410, "error in (no error)"=w409) -> ("pEnumSymbol"=w412:string, "error out"=w419:errorcluster)  [unwired: 7 in]
                      n184 = while {
                        tunnel: w413 -> [w428]
                        tunnel: w412 -> [w426]
                        tunnel: [w424] -> w411
                        i -> [w424]
                        stop <- w425 stop-if-true
                        n185 = Index Array(array=w428, index=w424) -> (element=w427:string)
                        n186 = Equal?(x=w427, y=w426) -> (x = y?=w425:bool)
                      }
                      n187 = property on="DeviceScanType" class="Ring (strict)"(error in=w419, "Value"=w411) -> (error out=w415:errorcluster)  [unwired: 1 in, 1 out]
                      n188 = property on="DeviceScanType" class="Ring (strict)"(error in=w415, "Strings []"=w413) -> (error out=w414:errorcluster)  [unwired: 1 in, 1 out]
                    }
                  }
                  n189 = case shown="True" w369 {
                    tunnel: [w376 w384] -> w363
                    tunnel: w366 -> [_ w379]
                    tunnel: w365 -> [w375 w380]
                    frame False {
                      n190 = property on="DeviceScanType 2" class="Ring (strict)"(error in=w375, "DisabledEnum"=T6."Disabled and Grayed Out" ("Disabled")) -> (error out=w376:errorcluster)  [unwired: 1 in, 1 out]
                    }
                    frame True {
                      w386 = "DeviceScanType" ("pFeatureName")
                      n191 = call "GetEnumFeatureEntryNum.vi"("handle"=w379, "pFeatureName"=w386, "error in (no error)"=w380) -> ("pEntryNum"=w390:u32, "error out"=w389:errorcluster)  [unwired: 7 in]
                      n192 = call "GetEnumFeatureEntrys.vi"("pFeatureName"=w386, "EntryNum"=w390, "handle"=w379, "error in (no error)"=w389) -> ("pLbEnumEntryList"=w391:string, "error out"=w378:errorcluster)  [unwired: 6 in]
                      n193 = for {
                        N: w390 -> [_]
                        shift-right: [w403] -> _
                        shift-left: 0 ("offset past token") -> [w404]
                        shift-right: [w401] -> _
                        shift-left: w391 -> [w402]
                        shift-right: [w399] -> w383
                        shift-left: string[] [] -> [w400]
                        n194 = Scan String For Tokens(6:string[] [":"] ("delimiters (\\s,\\t,\\r,\\n)"), 8:w404, 9:w402) -> (1:w398:string, 2:w403:i32, 3:w401:string)  [unwired: 3 in, 1 out]
                        n195 = Build Array (concatenate)(w400, w398) -> (w399:string[])
                      }
                      n196 = call "GetEnumFeatureSymbol.vi"("pFeatureName"=w386, "handle"=w379, "error in (no error)"=w378) -> ("pEnumSymbol"=w382:string, "error out"=w388:errorcluster)  [unwired: 7 in]
                      n197 = while {
                        tunnel: w383 -> [w397]
                        tunnel: w382 -> [w395]
                        tunnel: [w393] -> w381
                        i -> [w393]
                        stop <- w394 stop-if-true
                        n198 = Index Array(array=w397, index=w393) -> (element=w396:string)
                        n199 = Equal?(x=w396, y=w395) -> (x = y?=w394:bool)
                      }
                      n200 = property on="DeviceScanType 2" class="Ring (strict)"(error in=w388, "Value"=w381) -> (error out=w385:errorcluster)  [unwired: 1 in, 1 out]
                      n201 = property on="DeviceScanType 2" class="Ring (strict)"(error in=w385, "Strings []"=w383) -> (error out=w384:errorcluster)  [unwired: 1 in, 1 out]
                    }
                  }
                  n202 = Merge Errors(w364, w363) -> (w362:errorcluster)
                }
                frame "ExposureTime" {
                  n203 = call "GetDoubleFeatureValue.vi"("pFeatureName"="ExposureTime", "handle"=w445, "error in (no error)"=w446) -> ("pDoubleValue"=w448:dbl, "error out"=w449:errorcluster)  [unwired: 7 in]
                  n204 = call "GetDoubleFeatureValue.vi"("pFeatureName"="ExposureTime", "handle"=w441, "error in (no error)"=w440) -> ("pDoubleValue"=w443:dbl, "error out"=w444:errorcluster)  [unwired: 7 in]
                  n205 = property on="ExposureTime" class="DigNum (strict)"(error in=w449, "Value"=w448) -> (error out=w439:errorcluster)  [unwired: 1 in, 1 out]
                  n206 = property on="ExposureTime 2" class="DigNum (strict)"(error in=w444, "Value"=w443) -> (error out=w438:errorcluster)  [unwired: 1 in, 1 out]
                  n207 = Merge Errors(w439, w438) -> (w437:errorcluster)
                }
                frame "GainRaw" {
                  n208 = call "GetDoubleFeatureValue.vi"("pFeatureName"="GainRaw", "handle"=w458, "error in (no error)"=w459) -> ("pDoubleValue"=w460:dbl, "error out"=w461:errorcluster)  [unwired: 7 in]
                  n209 = call "GetDoubleFeatureValue.vi"("pFeatureName"="GainRaw", "handle"=w454, "error in (no error)"=w453) -> ("pDoubleValue"=w455:dbl, "error out"=w456:errorcluster)  [unwired: 7 in]
                  n210 = property on="GainRaw" class="DigNum (strict)"(error in=w461, "Value"=w460) -> (error out=w452:errorcluster)  [unwired: 1 in, 1 out]
                  n211 = property on="GainRaw 2" class="DigNum (strict)"(error in=w456, "Value"=w455) -> (error out=w451:errorcluster)  [unwired: 1 in, 1 out]
                  n212 = Merge Errors(w452, w451) -> (w450:errorcluster)
                }
                frame "Width" {
                  n213 = call "GetIntFeatureValue.vi"("pFeatureName"="Width", "handle"=w466, "error in (no error)"=w467) -> ("pIntValue"=w468:i64, "error out"=w469:errorcluster)  [unwired: 7 in]
                  n214 = call "GetIntFeatureValue.vi"("pFeatureName"="Width", "handle"=w471, "error in (no error)"=w472) -> ("pIntValue"=w473:i64, "error out"=w474:errorcluster)  [unwired: 7 in]
                  n215 = property on="Width 2" class="DigNum (strict)"(error in=w469, "Value"=w468) -> (error out=w465:errorcluster)  [unwired: 1 in, 1 out]
                  n216 = property on="Width" class="DigNum (strict)"(error in=w474, "Value"=w473) -> (error out=w464:errorcluster)  [unwired: 1 in, 1 out]
                  n217 = Merge Errors(w464, w465) -> (w463:errorcluster)
                }
                frame "Height" {
                  n218 = call "GetIntFeatureValue.vi"("pFeatureName"="Height", "handle"=w480, "error in (no error)"=w479) -> ("pIntValue"=w481:i64, "error out"=w482:errorcluster)  [unwired: 7 in]
                  n219 = call "GetIntFeatureValue.vi"("pFeatureName"="Height", "handle"=w484, "error in (no error)"=w485) -> ("pIntValue"=w486:i64, "error out"=w487:errorcluster)  [unwired: 7 in]
                  n220 = property on="Height 2" class="DigNum (strict)"(error in=w482, "Value"=w481) -> (error out=w477:errorcluster)  [unwired: 1 in, 1 out]
                  n221 = property on="Height" class="DigNum (strict)"(error in=w487, "Value"=w486) -> (error out=w478:errorcluster)  [unwired: 1 in, 1 out]
                  n222 = Merge Errors(w478, w477) -> (w476:errorcluster)
                }
                frame "PixelFormat" {
                  w500 = "PixelFormat" ("pFeatureName")
                  w514 = "PixelFormat" ("pFeatureName")
                  n223 = call "GetEnumFeatureEntryNum.vi"("handle"=w507, "pFeatureName"=w514, "error in (no error)"=w506) -> ("pEntryNum"=w516:u32, "error out"=w519:errorcluster)  [unwired: 7 in]
                  n224 = call "GetEnumFeatureEntryNum.vi"("handle"=w492, "pFeatureName"=w500, "error in (no error)"=w493) -> ("pEntryNum"=w502:u32, "error out"=w505:errorcluster)  [unwired: 7 in]
                  n225 = call "GetEnumFeatureEntrys.vi"("pFeatureName"=w514, "EntryNum"=w516, "handle"=w507, "error in (no error)"=w519) -> ("pLbEnumEntryList"=w518:string, "error out"=w513:errorcluster)  [unwired: 6 in]
                  n226 = call "GetEnumFeatureEntrys.vi"("pFeatureName"=w500, "EntryNum"=w502, "handle"=w492, "error in (no error)"=w505) -> ("pLbEnumEntryList"=w504:string, "error out"=w499:errorcluster)  [unwired: 6 in]
                  n227 = for {
                    N: w516 -> [_]
                    shift-right: [w543] -> _
                    shift-left: 0 ("offset past token") -> [w544]
                    shift-right: [w541] -> _
                    shift-left: w518 -> [w542]
                    shift-right: [w539] -> w509
                    shift-left: string[] [] -> [w540]
                    n228 = Scan String For Tokens(6:string[] [":"] ("delimiters (\\s,\\t,\\r,\\n)"), 8:w544, 9:w542) -> (1:w538:string, 2:w543:i32, 3:w541:string)  [unwired: 3 in, 1 out]
                    n229 = Build Array (concatenate)(w540, w538) -> (w539:string[])
                  }
                  n230 = for {
                    N: w502 -> [_]
                    shift-right: [w530] -> _
                    shift-left: 0 ("offset past token") -> [w531]
                    shift-right: [w528] -> _
                    shift-left: w504 -> [w529]
                    shift-right: [w526] -> w495
                    shift-left: string[] [] -> [w527]
                    n231 = Scan String For Tokens(6:string[] [":"] ("delimiters (\\s,\\t,\\r,\\n)"), 8:w531, 9:w529) -> (1:w525:string, 2:w530:i32, 3:w528:string)  [unwired: 3 in, 1 out]
                    n232 = Build Array (concatenate)(w527, w525) -> (w526:string[])
                  }
                  n233 = property on="PixelFormat" class="Ring (strict)"(error in=w513, "Strings []"=w509) -> (error out=w512:errorcluster)  [unwired: 1 in, 1 out]
                  n234 = property on="PixelFormat 2" class="Ring (strict)"(error in=w499, "Strings []"=w495) -> (error out=w498:errorcluster)  [unwired: 1 in, 1 out]
                  n235 = call "GetEnumFeatureSymbol.vi"("pFeatureName"=w514, "handle"=w507, "error in (no error)"=w512) -> ("pEnumSymbol"=w510:string, "error out"=w511:errorcluster)  [unwired: 7 in]
                  n236 = call "GetEnumFeatureSymbol.vi"("pFeatureName"=w500, "handle"=w492, "error in (no error)"=w498) -> ("pEnumSymbol"=w496:string, "error out"=w497:errorcluster)  [unwired: 7 in]
                  n237 = while {
                    tunnel: w509 -> [w537]
                    tunnel: w510 -> [w535]
                    tunnel: [w533] -> w508
                    i -> [w533]
                    stop <- w534 stop-if-true
                    n238 = Index Array(array=w537, index=w533) -> (element=w536:string)
                    n239 = Equal?(x=w536, y=w535) -> (x = y?=w534:bool)
                  }
                  n240 = while {
                    tunnel: w495 -> [w524]
                    tunnel: w496 -> [w522]
                    tunnel: [w520] -> w494
                    i -> [w520]
                    stop <- w521 stop-if-true
                    n241 = Index Array(array=w524, index=w520) -> (element=w523:string)
                    n242 = Equal?(x=w523, y=w522) -> (x = y?=w521:bool)
                  }
                  n243 = property on="PixelFormat" class="Ring (strict)"(error in=w511, "Value"=w508) -> (error out=w491:errorcluster)  [unwired: 1 in, 1 out]
                  n244 = property on="PixelFormat 2" class="Ring (strict)"(error in=w497, "Value"=w494) -> (error out=w490:errorcluster)  [unwired: 1 in, 1 out]
                  n245 = Merge Errors(w491, w490) -> (w489:errorcluster)
                }
                frame "TriggerSource" {
                  w551 = "TriggerSource" ("pFeatureName")
                  n246 = call "GetEnumFeatureEntryNum.vi"("handle"=w552, "pFeatureName"=w551, "error in (no error)"=w553) -> ("pEntryNum"=w557:u32, "error out"=w560:errorcluster)  [unwired: 7 in]
                  n247 = call "GetEnumFeatureEntrys.vi"("pFeatureName"=w551, "EntryNum"=w557, "handle"=w552, "error in (no error)"=w560) -> ("pLbEnumEntryList"=w559:string, "error out"=w555:errorcluster)  [unwired: 6 in]
                  n248 = for {
                    N: w557 -> [_]
                    shift-right: [w571] -> _
                    shift-left: 0 ("offset past token") -> [w572]
                    shift-right: [w569] -> _
                    shift-left: w559 -> [w570]
                    shift-right: [w567] -> w548
                    shift-left: string[] [] -> [w568]
                    n249 = Scan String For Tokens(6:string[] [":"] ("delimiters (\\s,\\t,\\r,\\n)"), 8:w572, 9:w570) -> (1:w566:string, 2:w571:i32, 3:w569:string)  [unwired: 3 in, 1 out]
                    n250 = Build Array (concatenate)(w568, w566) -> (w567:string[])
                  }
                  n251 = property on="TriggerSource" class="Ring (strict)"(error in=w555, "Strings []"=w548) -> (error out=w554:errorcluster)  [unwired: 1 in, 1 out]
                  n252 = call "GetEnumFeatureSymbol.vi"("pFeatureName"=w551, "handle"=w552, "error in (no error)"=w554) -> ("pEnumSymbol"=w547:string, "error out"=w550:errorcluster)  [unwired: 7 in]
                  n253 = while {
                    tunnel: w548 -> [w565]
                    tunnel: w547 -> [w563]
                    tunnel: [w561] -> w546
                    i -> [w561]
                    stop <- w562 stop-if-true
                    n254 = Index Array(array=w565, index=w561) -> (element=w564:string)
                    n255 = Equal?(x=w564, y=w563) -> (x = y?=w562:bool)
                  }
                  n256 = property on="TriggerSource" class="Ring (strict)"(error in=w550, "Value"=w546) -> (error out=w549:errorcluster)  [unwired: 1 in, 1 out]
                }
                frame "ExposureAuto" {
                  n257 = property on="DeviceInterfaceType" class="Ring (strict)"() -> ("Value"=w581:u16)  [unwired: 2 in, 2 out]
                  n258 = property on="DeviceInterfaceType" class="Ring (strict)"() -> ("Value"=w584:u16)  [unwired: 2 in, 2 out]
                  n259 = Not Equal?(x=w581, y=u16 3) -> (x != y?=w579:bool)
                  n260 = Not Equal?(x=w584, y=u16 3) -> (x != y?=w582:bool)
                  n261 = case shown="False" w579 {
                    tunnel: w578 -> [w588 w596]
                    tunnel: w577 -> [_ w595]
                    tunnel: [w587 w593] -> w575
                    frame False {
                      n262 = property on="ExposureAuto 2" class="Ring (strict)"(error in=w588, "DisabledEnum"=T6."Disabled and Grayed Out" ("Disabled")) -> (error out=w587:errorcluster)  [unwired: 1 in, 1 out]
                    }
                    frame True {
                      w604 = "ExposureAuto" ("pFeatureName")
                      n263 = call "GetEnumFeatureEntryNum.vi"("handle"=w595, "pFeatureName"=w604, "error in (no error)"=w596) -> ("pEntryNum"=w600:u32, "error out"=w597:errorcluster)  [unwired: 7 in]
                      n264 = call "GetEnumFeatureEntrys.vi"("pFeatureName"=w604, "EntryNum"=w600, "handle"=w595, "error in (no error)"=w597) -> ("pLbEnumEntryList"=w598:string, "error out"=w602:errorcluster)  [unwired: 6 in]
                      n265 = for {
                        N: w600 -> [_]
                        shift-right: [w615] -> _
                        shift-left: 0 ("offset past token") -> [w616]
                        shift-right: [w613] -> _
                        shift-left: w598 -> [w614]
                        shift-right: [w611] -> w592
                        shift-left: string[] [] -> [w612]
                        n266 = Scan String For Tokens(6:string[] [":"] ("delimiters (\\s,\\t,\\r,\\n)"), 8:w616, 9:w614) -> (1:w610:string, 2:w615:i32, 3:w613:string)  [unwired: 3 in, 1 out]
                        n267 = Build Array (concatenate)(w612, w610) -> (w611:string[])
                      }
                      n268 = property on="ExposureAuto 2" class="Ring (strict)"(error in=w602, "Strings []"=w592) -> (error out=w603:errorcluster)  [unwired: 1 in, 1 out]
                      n269 = call "GetEnumFeatureSymbol.vi"("pFeatureName"=w604, "handle"=w595, "error in (no error)"=w603) -> ("pEnumSymbol"=w591:string, "error out"=w594:errorcluster)  [unwired: 7 in]
                      n270 = while {
                        tunnel: w592 -> [w609]
                        tunnel: w591 -> [w607]
                        tunnel: [w605] -> w590
                        i -> [w605]
                        stop <- w606 stop-if-true
                        n271 = Index Array(array=w609, index=w605) -> (element=w608:string)
                        n272 = Equal?(x=w608, y=w607) -> (x = y?=w606:bool)
                      }
                      n273 = property on="ExposureAuto 2" class="Ring (strict)"(error in=w594, "Value"=w590) -> (error out=w593:errorcluster)  [unwired: 1 in, 1 out]
                    }
                  }
                  n274 = case shown="False" w582 {
                    tunnel: w586 -> [w619 w627]
                    tunnel: w585 -> [_ w626]
                    tunnel: [w618 w624] -> w576
                    frame False {
                      n275 = property on="ExposureAuto" class="Ring (strict)"(error in=w619, "DisabledEnum"=T6."Disabled and Grayed Out" ("Disabled")) -> (error out=w618:errorcluster)  [unwired: 1 in, 1 out]
                    }
                    frame True {
                      w635 = "ExposureAuto" ("pFeatureName")
                      n276 = call "GetEnumFeatureEntryNum.vi"("handle"=w626, "pFeatureName"=w635, "error in (no error)"=w627) -> ("pEntryNum"=w631:u32, "error out"=w628:errorcluster)  [unwired: 7 in]
                      n277 = call "GetEnumFeatureEntrys.vi"("pFeatureName"=w635, "EntryNum"=w631, "handle"=w626, "error in (no error)"=w628) -> ("pLbEnumEntryList"=w629:string, "error out"=w633:errorcluster)  [unwired: 6 in]
                      n278 = for {
                        N: w631 -> [_]
                        shift-right: [w646] -> _
                        shift-left: 0 ("offset past token") -> [w647]
                        shift-right: [w644] -> _
                        shift-left: w629 -> [w645]
                        shift-right: [w642] -> w623
                        shift-left: string[] [] -> [w643]
                        n279 = Scan String For Tokens(6:string[] [":"] ("delimiters (\\s,\\t,\\r,\\n)"), 8:w647, 9:w645) -> (1:w641:string, 2:w646:i32, 3:w644:string)  [unwired: 3 in, 1 out]
                        n280 = Build Array (concatenate)(w643, w641) -> (w642:string[])
                      }
                      n281 = property on="ExposureAuto" class="Ring (strict)"(error in=w633, "Strings []"=w623) -> (error out=w634:errorcluster)  [unwired: 1 in, 1 out]
                      n282 = call "GetEnumFeatureSymbol.vi"("pFeatureName"=w635, "handle"=w626, "error in (no error)"=w634) -> ("pEnumSymbol"=w622:string, "error out"=w625:errorcluster)  [unwired: 7 in]
                      n283 = while {
                        tunnel: w623 -> [w640]
                        tunnel: w622 -> [w638]
                        tunnel: [w636] -> w621
                        i -> [w636]
                        stop <- w637 stop-if-true
                        n284 = Index Array(array=w640, index=w636) -> (element=w639:string)
                        n285 = Equal?(x=w639, y=w638) -> (x = y?=w637:bool)
                      }
                      n286 = property on="ExposureAuto" class="Ring (strict)"(error in=w625, "Value"=w621) -> (error out=w624:errorcluster)  [unwired: 1 in, 1 out]
                    }
                  }
                  n287 = Merge Errors(w576, w575) -> (w574:errorcluster)
                }
              }
            }
            n288 = Merge Errors(w354) -> (w353:errorcluster)
          }
        }
      }
    }
    n289 = local read "QuitFlag"() -> (w321:bool)
    n290 = local write "error out"(w323) -> ()
    n291 = Wait (ms)(milliseconds to wait=u32 2000) -> ()  [unwired: 1 out]
  }
  n292 = while {
    tunnel: w1 -> [w652]
    stop <- w650 stop-if-true
    # "属性值改变"
    n293 = event shown="[3] \"ExposureTime\": Value Change" {
      selector: _ -> [_ _ _ _ _ _ _ _ _ _ _ _ _ _ _ _]
      dyn-events: _ -> [_ _ _ _ _ _ _ _ _ _ _ _ _ _ _ _]
      timeout: _ -> [_ _ _ _ _ _ _ _ _ _ _ _ _ _ _ _]
      tunnel: w652 -> [_ w660 w679 w708 w728 w757 w778 w807 w830 w861 w883 w914 w938 w962 w1030 w1055]
      tunnel: [errorcluster {FALSE, 0, "Timeout"} w659 _ w709 _ w758 w777 w808 w829 w862 _ w915 _ w970 w1031 _] -> w651
      event Timeout {
        n294 = event-data() -> ()  [unwired: 1 in, 3 out]
      }
      event "DeviceScanType": Value Change {
        n295 = event-data() -> ()  [unwired: 1 in, 6 out]
        n296 = local read "hIFDev"() -> (w655:i64)
        n297 = local read "hDev"() -> (w654:i64)
        n298 = Not Equal To 0?(x=w655) -> (x != 0?=w658:bool)
        n299 = Not Equal To 0?(x=w654) -> (x != 0?=w657:bool)
        n300 = And(x=w658, y=w657) -> (x .and. y?=w656:bool)
        n301 = case shown="True" w656 {
          tunnel: w660 -> [_ w672]
          tunnel: [errorcluster {"status"=FALSE, "code"=0, "source"="设备句柄为空"} ("error in") w664] -> w659
          tunnel: w655 -> [_ w662]
          tunnel: w654 -> [_ w663]
          frame False {
          }
          frame True {
            n302 = call "IsOpenInterface.vi"("interface handle"=w662, "error in (no error)"=w672) -> ("return type"=w668:i8, "error out"=w671:errorcluster)  [unwired: 8 in]
            n303 = call "IsDeviceOpen.vi"("dev handle"=w663, "error in (no error)"=w671) -> ("return type"=w669:i8, "error out"=w670:errorcluster)  [unwired: 8 in]
            n304 = Not Equal To 0?(x=w668) -> (x != 0?=w665:bool)
            n305 = Not Equal To 0?(x=w669) -> (x != 0?=w666:bool)
            n306 = And(x=w666, y=w665) -> (x .and. y?=w667:bool)
            n307 = case shown="True" w667 {
              tunnel: w670 -> [w673 w678]
              tunnel: [w673 w677] -> w664
              tunnel: w662 -> [_ w674]
              frame False {
              }
              frame True {
                n308 = property on="DeviceScanType" class="Ring (strict)"() -> ("RingText.Text"=w675:string)  [unwired: 2 in, 2 out]
                n309 = call "SetEnumFeatureSymbol.vi"("pEnumSymbol"=w675, "pFeatureName"="DeviceScanType", "handle"=w674, "error in (no error)"=w678) -> ("error out"=w677:errorcluster)  [unwired: 6 in, 1 out]
              }
            }
          }
        }
      }
      event "DeviceScanType 2": Value Change {
        n310 = event-data() -> ()  [unwired: 1 in, 6 out]
        n311 = local read "hIFDev 2"() -> (w681:i64)
        n312 = local read "hDev 2"() -> (w680:i64)
        n313 = Not Equal To 0?(x=w681) -> (x != 0?=w684:bool)
        n314 = Not Equal To 0?(x=w680) -> (x != 0?=w683:bool)
        n315 = And(x=w684, y=w683) -> (x .and. y?=w682:bool)
        n316 = case shown="True" w682 {
          tunnel: w679 -> [_ w696]
          tunnel: [errorcluster {"status"=FALSE, "code"=0, "source"="设备句柄为空"} ("error in") w688] -> _
          tunnel: w681 -> [_ w686]
          tunnel: w680 -> [_ w687]
          frame False {
          }
          frame True {
            n317 = call "IsOpenInterface.vi"("interface handle"=w686, "error in (no error)"=w696) -> ("return type"=w692:i8, "error out"=w695:errorcluster)  [unwired: 8 in]
            n318 = call "IsDeviceOpen.vi"("dev handle"=w687, "error in (no error)"=w695) -> ("return type"=w693:i8, "error out"=w694:errorcluster)  [unwired: 8 in]
            n319 = Not Equal To 0?(x=w692) -> (x != 0?=w689:bool)
            n320 = Not Equal To 0?(x=w693) -> (x != 0?=w690:bool)
            n321 = And(x=w690, y=w689) -> (x .and. y?=w691:bool)
            n322 = case shown="True" w691 {
              tunnel: w694 -> [w697 w702]
              tunnel: [w697 w701] -> w688
              tunnel: w686 -> [_ w698]
              frame False {
              }
              frame True {
                n323 = property on="DeviceScanType 2" class="Ring (strict)"() -> ("RingText.Text"=w699:string)  [unwired: 2 in, 2 out]
                n324 = call "SetEnumFeatureSymbol.vi"("pEnumSymbol"=w699, "pFeatureName"="DeviceScanType", "handle"=w698, "error in (no error)"=w702) -> ("error out"=w701:errorcluster)  [unwired: 6 in, 1 out]
              }
            }
          }
        }
      }
      event "ExposureTime": Value Change {
        n325 = event-data() -> ()  [unwired: 1 in, 6 out]
        n326 = local read "hDev"() -> (w706:i64)
        n327 = local read "hIFDev"() -> (w707:i64)
        n328 = Not Equal To 0?(x=w707) -> (x != 0?=w705:bool)
        n329 = Not Equal To 0?(x=w706) -> (x != 0?=w704:bool)
        n330 = And(x=w705, y=w704) -> (x .and. y?=w703:bool)
        n331 = case shown="True" w703 {
          tunnel: [errorcluster {FALSE, 0, "设备句柄为空"} w712] -> w709
          tunnel: w707 -> [_ w716]
          tunnel: w706 -> [_ w713]
          tunnel: w708 -> [_ w711]
          frame False {
          }
          frame True {
            n332 = call "IsOpenInterface.vi"("interface handle"=w716, "error in (no error)"=w711) -> ("return type"=w719:i8, "error out"=w717:errorcluster)  [unwired: 8 in]
            n333 = Not Equal To 0?(x=w719) -> (x != 0?=w721:bool)
            n334 = call "IsDeviceOpen.vi"("dev handle"=w713, "error in (no error)"=w717) -> ("return type"=w718:i8, "error out"=w714:errorcluster)  [unwired: 8 in]
            n335 = Not Equal To 0?(x=w718) -> (x != 0?=w720:bool)
            n336 = And(x=w720, y=w721) -> (x .and. y?=w715:bool)
            n337 = case shown="True" w715 {
              tunnel: w714 -> [w722 w727]
              tunnel: w713 -> [_ w726]
              tunnel: [w722 w723] -> w712
              frame False {
              }
              frame True {
                n338 = property on="ExposureTime" class="DigNum (strict)"() -> ("Value"=w724:dbl)  [unwired: 2 in, 2 out]
                n339 = call "SetDoubleFeatureValue.vi"("doubleValue"=w724, "pFeatureName"="ExposureTime", "handle"=w726, "error in (no error)"=w727) -> ("error out"=w723:errorcluster)  [unwired: 7 in]
              }
            }
          }
        }
      }
      event "ExposureTime 2": Value Change {
        n340 = event-data() -> ()  [unwired: 1 in, 6 out]
        n341 = local read "hIFDev 2"() -> (w729:i64)
        n342 = local read "hDev 2"() -> (w730:i64)
        n343 = Not Equal To 0?(x=w729) -> (x != 0?=w733:bool)
        n344 = Not Equal To 0?(x=w730) -> (x != 0?=w732:bool)
        n345 = And(x=w733, y=w732) -> (x .and. y?=w731:bool)
        n346 = case shown="True" w731 {
          tunnel: [errorcluster {FALSE, 0, "设备句柄为空"} w736] -> _
          tunnel: w729 -> [_ w740]
          tunnel: w730 -> [_ w737]
          tunnel: w728 -> [_ w735]
          frame False {
          }
          frame True {
            n347 = call "IsOpenInterface.vi"("interface handle"=w740, "error in (no error)"=w735) -> ("return type"=w743:i8, "error out"=w741:errorcluster)  [unwired: 8 in]
            n348 = Not Equal To 0?(x=w743) -> (x != 0?=w745:bool)
            n349 = call "IsDeviceOpen.vi"("dev handle"=w737, "error in (no error)"=w741) -> ("return type"=w742:i8, "error out"=w738:errorcluster)  [unwired: 8 in]
            n350 = Not Equal To 0?(x=w742) -> (x != 0?=w744:bool)
            n351 = And(x=w744, y=w745) -> (x .and. y?=w739:bool)
            n352 = case shown="True" w739 {
              tunnel: w738 -> [w746 w751]
              tunnel: w737 -> [_ w750]
              tunnel: [w746 w747] -> w736
              frame False {
              }
              frame True {
                n353 = property on="ExposureTime 2" class="DigNum (strict)"() -> ("Value"=w748:dbl)  [unwired: 2 in, 2 out]
                n354 = call "SetDoubleFeatureValue.vi"("doubleValue"=w748, "pFeatureName"="ExposureTime", "handle"=w750, "error in (no error)"=w751) -> ("error out"=w747:errorcluster)  [unwired: 7 in]
              }
            }
          }
        }
      }
      event "GainRaw": Value Change {
        n355 = event-data() -> ()  [unwired: 1 in, 6 out]
        n356 = local read "hIFDev"() -> (w755:i64)
        n357 = local read "hDev"() -> (w754:i64)
        n358 = Not Equal To 0?(x=w755) -> (x != 0?=w752:bool)
        n359 = Not Equal To 0?(x=w754) -> (x != 0?=w753:bool)
        n360 = And(x=w752, y=w753) -> (x .and. y?=w756:bool)
        n361 = case shown="True" w756 {
          tunnel: w755 -> [_ w764]
          tunnel: w754 -> [_ w761]
          tunnel: [errorcluster {FALSE, 0, "设备句柄为空"} w762] -> w758
          tunnel: w757 -> [_ w760]
          frame False {
          }
          frame True {
            n362 = call "IsOpenInterface.vi"("interface handle"=w764, "error in (no error)"=w760) -> ("return type"=w768:i8, "error out"=w766:errorcluster)  [unwired: 8 in]
            n363 = Not Equal To 0?(x=w768) -> (x != 0?=w770:bool)
            n364 = call "IsDeviceOpen.vi"("dev handle"=w761, "error in (no error)"=w766) -> ("return type"=w767:i8, "error out"=w763:errorcluster)  [unwired: 8 in]
            n365 = Not Equal To 0?(x=w767) -> (x != 0?=w769:bool)
            n366 = And(x=w769, y=w770) -> (x .and. y?=w765:bool)
            n367 = case shown="True" w765 {
              tunnel: w763 -> [w771 w776]
              tunnel: [w771 w772] -> w762
              tunnel: w761 -> [_ w775]
              frame False {
              }
              frame True {
                n368 = property on="GainRaw" class="DigNum (strict)"() -> ("Value"=w773:dbl)  [unwired: 2 in, 2 out]
                n369 = call "SetDoubleFeatureValue.vi"("doubleValue"=w773, "pFeatureName"="GainRaw", "handle"=w775, "error in (no error)"=w776) -> ("error out"=w772:errorcluster)  [unwired: 7 in]
              }
            }
          }
        }
      }
      event "GainRaw 2": Value Change {
        n370 = event-data() -> ()  [unwired: 1 in, 6 out]
        n371 = local read "hIFDev 2"() -> (w780:i64)
        n372 = local read "hDev 2"() -> (w779:i64)
        n373 = Not Equal To 0?(x=w780) -> (x != 0?=w781:bool)
        n374 = Not Equal To 0?(x=w779) -> (x != 0?=w782:bool)
        n375 = And(x=w781, y=w782) -> (x .and. y?=w783:bool)
        n376 = case shown="True" w783 {
          tunnel: w780 -> [_ w789]
          tunnel: w779 -> [_ w786]
          tunnel: [errorcluster {FALSE, 0, "设备句柄为空"} w787] -> w777
          tunnel: w778 -> [_ w785]
          frame False {
          }
          frame True {
            n377 = call "IsOpenInterface.vi"("interface handle"=w789, "error in (no error)"=w785) -> ("return type"=w793:i8, "error out"=w791:errorcluster)  [unwired: 8 in]
            n378 = Not Equal To 0?(x=w793) -> (x != 0?=w795:bool)
            n379 = call "IsDeviceOpen.vi"("dev handle"=w786, "error in (no error)"=w791) -> ("return type"=w792:i8, "error out"=w788:errorcluster)  [unwired: 8 in]
            n380 = Not Equal To 0?(x=w792) -> (x != 0?=w794:bool)
            n381 = And(x=w794, y=w795) -> (x .and. y?=w790:bool)
            n382 = case shown="True" w790 {
              tunnel: w788 -> [w796 w801]
              tunnel: [w796 w797] -> w787
              tunnel: w786 -> [_ w800]
              frame False {
              }
              frame True {
                n383 = property on="GainRaw 2" class="DigNum (strict)"() -> ("Value"=w798:dbl)  [unwired: 2 in, 2 out]
                n384 = call "SetDoubleFeatureValue.vi"("doubleValue"=w798, "pFeatureName"="GainRaw", "handle"=w800, "error in (no error)"=w801) -> ("error out"=w797:errorcluster)  [unwired: 7 in]
              }
            }
          }
        }
      }
      event "Width": Value Change {
        n385 = event-data() -> ()  [unwired: 1 in, 6 out]
        n386 = local read "hIFDev"() -> (w805:i64)
        n387 = local read "hDev"() -> (w804:i64)
        n388 = Not Equal To 0?(x=w805) -> (x != 0?=w803:bool)
        n389 = Not Equal To 0?(x=w804) -> (x != 0?=w802:bool)
        n390 = And(x=w803, y=w802) -> (x .and. y?=w806:bool)
        n391 = case shown="True" w806 {
          tunnel: [errorcluster {"status"=FALSE, "code"=0, "source"="设备句柄为空"} ("error in") w814] -> w808
          tunnel: w805 -> [_ w810]
          tunnel: w804 -> [_ w812]
          tunnel: w807 -> [_ w811]
          frame False {
          }
          frame True {
            n392 = call "IsOpenInterface.vi"("interface handle"=w810, "error in (no error)"=w811) -> ("return type"=w818:i8, "error out"=w820:errorcluster)  [unwired: 8 in]
            n393 = Not Equal To 0?(x=w818) -> (x != 0?=w816:bool)
            n394 = call "IsDeviceOpen.vi"("dev handle"=w812, "error in (no error)"=w820) -> ("return type"=w819:i8, "error out"=w815:errorcluster)  [unwired: 8 in]
            n395 = Not Equal To 0?(x=w819) -> (x != 0?=w817:bool)
            n396 = And(x=w817, y=w816) -> (x .and. y?=w813:bool)
            n397 = case shown="True" w813 {
              tunnel: w815 -> [w821 w827]
              tunnel: [w821 w825] -> w814
              tunnel: w812 -> [_ w828]
              tunnel: w810 -> [_ w824]
              frame False {
              }
              frame True {
                w823 = "Width" ("pFeatureName")
                n398 = property on="Width" class="DigNum (strict)"() -> ("Value"=w822:i32)  [unwired: 2 in, 2 out]
                n399 = call "SetIntFeatureValue.vi"("intValue"=w822, "pFeatureName"=w823, "handle"=w828, "error in (no error)"=w827) -> ("error out"=w826:errorcluster)  [unwired: 7 in]
                n400 = call "SetIntFeatureValue.vi"("intValue"=w822, "pFeatureName"=w823, "handle"=w824, "error in (no error)"=w826) -> ("error out"=w825:errorcluster)  [unwired: 7 in]
              }
            }
          }
        }
      }
      event "Width 2": Value Change {
        n401 = event-data() -> ()  [unwired: 1 in, 6 out]
        n402 = local read "hIFDev 2"() -> (w832:i64)
        n403 = local read "hDev 2"() -> (w831:i64)
        n404 = Not Equal To 0?(x=w832) -> (x != 0?=w834:bool)
        n405 = Not Equal To 0?(x=w831) -> (x != 0?=w833:bool)
        n406 = And(x=w834, y=w833) -> (x .and. y?=w835:bool)
        n407 = case shown="True" w835 {
          tunnel: [errorcluster {"status"=FALSE, "code"=0, "source"="设备句柄为空"} ("error in") w841] -> w829
          tunnel: w832 -> [_ w838]
          tunnel: w831 -> [_ w839]
          tunnel: w830 -> [_ w837]
          frame False {
          }
          frame True {
            n408 = call "IsOpenInterface.vi"("interface handle"=w838, "error in (no error)"=w837) -> ("return type"=w845:i8, "error out"=w847:errorcluster)  [unwired: 8 in]
            n409 = Not Equal To 0?(x=w845) -> (x != 0?=w843:bool)
            n410 = call "IsDeviceOpen.vi"("dev handle"=w839, "error in (no error)"=w847) -> ("return type"=w846:i8, "error out"=w842:errorcluster)  [unwired: 8 in]
            n411 = Not Equal To 0?(x=w846) -> (x != 0?=w844:bool)
            n412 = And(x=w844, y=w843) -> (x .and. y?=w840:bool)
            n413 = case shown="True" w840 {
              tunnel: w842 -> [w848 w854]
              tunnel: [w848 w852] -> w841
              tunnel: w839 -> [_ w855]
              tunnel: w838 -> [_ w851]
              frame False {
              }
              frame True {
                w850 = "Width" ("pFeatureName")
                n414 = property on="Width 2" class="DigNum (strict)"() -> ("Value"=w849:i32)  [unwired: 2 in, 2 out]
                n415 = call "SetIntFeatureValue.vi"("intValue"=w849, "pFeatureName"=w850, "handle"=w855, "error in (no error)"=w854) -> ("error out"=w853:errorcluster)  [unwired: 7 in]
                n416 = call "SetIntFeatureValue.vi"("intValue"=w849, "pFeatureName"=w850, "handle"=w851, "error in (no error)"=w853) -> ("error out"=w852:errorcluster)  [unwired: 7 in]
              }
            }
          }
        }
      }
      event "Height": Value Change {
        n417 = event-data() -> ()  [unwired: 1 in, 6 out]
        n418 = local read "hIFDev"() -> (w857:i64)
        n419 = local read "hDev"() -> (w856:i64)
        n420 = Not Equal To 0?(x=w857) -> (x != 0?=w859:bool)
        n421 = Not Equal To 0?(x=w856) -> (x != 0?=w858:bool)
        n422 = And(x=w859, y=w858) -> (x .and. y?=w860:bool)
        n423 = case shown="True" w860 {
          tunnel: [errorcluster {FALSE, 0, "设备句柄为空"} w867] -> w862
          tunnel: w857 -> [_ w864]
          tunnel: w856 -> [_ w866]
          tunnel: w861 -> [_ w865]
          frame False {
          }
          frame True {
            n424 = call "IsOpenInterface.vi"("interface handle"=w864, "error in (no error)"=w865) -> ("return type"=w872:i8, "error out"=w870:errorcluster)  [unwired: 8 in]
            n425 = Not Equal To 0?(x=w872) -> (x != 0?=w874:bool)
            n426 = call "IsDeviceOpen.vi"("dev handle"=w866, "error in (no error)"=w870) -> ("return type"=w871:i8, "error out"=w868:errorcluster)  [unwired: 8 in]
            n427 = Not Equal To 0?(x=w871) -> (x != 0?=w873:bool)
            n428 = And(x=w873, y=w874) -> (x .and. y?=w869:bool)
            n429 = case shown="True" w869 {
              tunnel: w868 -> [w875 w882]
              tunnel: [w875 w876] -> w867
              tunnel: w866 -> [_ w881]
              tunnel: w864 -> [_ w877]
              frame False {
              }
              frame True {
                w879 = "Height" ("pFeatureName")
                n430 = property on="Height" class="DigNum (strict)"() -> ("Value"=w878:i32)  [unwired: 2 in, 2 out]
                n431 = call "SetIntFeatureValue.vi"("intValue"=w878, "pFeatureName"=w879, "handle"=w881, "error in (no error)"=w882) -> ("error out"=w880:errorcluster)  [unwired: 7 in]
                n432 = call "SetIntFeatureValue.vi"("intValue"=w878, "pFeatureName"=w879, "handle"=w877, "error in (no error)"=w880) -> ("error out"=w876:errorcluster)  [unwired: 7 in]
              }
            }
          }
        }
      }
      event "Height 2": Value Change {
        n433 = event-data() -> ()  [unwired: 1 in, 6 out]
        n434 = local read "hIFDev 2"() -> (w885:i64)
        n435 = local read "hDev 2"() -> (w884:i64)
        n436 = Not Equal To 0?(x=w885) -> (x != 0?=w887:bool)
        n437 = Not Equal To 0?(x=w884) -> (x != 0?=w886:bool)
        n438 = And(x=w887, y=w886) -> (x .and. y?=w888:bool)
        n439 = case shown="True" w888 {
          tunnel: [errorcluster {FALSE, 0, "设备句柄为空"} w893] -> _
          tunnel: w885 -> [_ w890]
          tunnel: w884 -> [_ w892]
          tunnel: w883 -> [_ w891]
          frame False {
          }
          frame True {
            n440 = call "IsOpenInterface.vi"("interface handle"=w890, "error in (no error)"=w891) -> ("return type"=w898:i8, "error out"=w896:errorcluster)  [unwired: 8 in]
            n441 = Not Equal To 0?(x=w898) -> (x != 0?=w900:bool)
            n442 = call "IsDeviceOpen.vi"("dev handle"=w892, "error in (no error)"=w896) -> ("return type"=w897:i8, "error out"=w894:errorcluster)  [unwired: 8 in]
            n443 = Not Equal To 0?(x=w897) -> (x != 0?=w899:bool)
            n444 = And(x=w899, y=w900) -> (x .and. y?=w895:bool)
            n445 = case shown="True" w895 {
              tunnel: w894 -> [w901 w908]
              tunnel: [w901 w902] -> w893
              tunnel: w892 -> [_ w907]
              tunnel: w890 -> [_ w903]
              frame False {
              }
              frame True {
                w905 = "Height" ("pFeatureName")
                n446 = property on="Height 2" class="DigNum (strict)"() -> ("Value"=w904:i32)  [unwired: 2 in, 2 out]
                n447 = call "SetIntFeatureValue.vi"("intValue"=w904, "pFeatureName"=w905, "handle"=w907, "error in (no error)"=w908) -> ("error out"=w906:errorcluster)  [unwired: 7 in]
                n448 = call "SetIntFeatureValue.vi"("intValue"=w904, "pFeatureName"=w905, "handle"=w903, "error in (no error)"=w906) -> ("error out"=w902:errorcluster)  [unwired: 7 in]
              }
            }
          }
        }
      }
      event "PixelFormat": Value Change {
        n449 = event-data() -> ()  [unwired: 1 in, 6 out]
        n450 = local read "hIFDev"() -> (w912:i64)
        n451 = local read "hDev"() -> (w911:i64)
        n452 = Not Equal To 0?(x=w912) -> (x != 0?=w909:bool)
        n453 = Not Equal To 0?(x=w911) -> (x != 0?=w910:bool)
        n454 = And(x=w909, y=w910) -> (x .and. y?=w913:bool)
        n455 = case shown="True" w913 {
          tunnel: [errorcluster {FALSE, 0, "设备句柄为空"} w920] -> w915
          tunnel: w912 -> [_ w917]
          tunnel: w911 -> [_ w919]
          tunnel: w914 -> [_ w918]
          frame False {
          }
          frame True {
            n456 = call "IsOpenInterface.vi"("interface handle"=w917, "error in (no error)"=w918) -> ("return type"=w926:i8, "error out"=w923:errorcluster)  [unwired: 8 in]
            n457 = Not Equal To 0?(x=w926) -> (x != 0?=w924:bool)
            n458 = call "IsDeviceOpen.vi"("dev handle"=w919, "error in (no error)"=w923) -> ("return type"=w927:i8, "error out"=w921:errorcluster)  [unwired: 8 in]
            n459 = Not Equal To 0?(x=w927) -> (x != 0?=w925:bool)
            n460 = And(x=w925, y=w924) -> (x .and. y?=w922:bool)
            n461 = case shown="True" w922 {
              tunnel: w921 -> [w928 w935]
              tunnel: [w928 w929] -> w920
              tunnel: w919 -> [_ w934]
              tunnel: w917 -> [_ w930]
              frame False {
              }
              frame True {
                w932 = "PixelFormat" ("pFeatureName")
                n462 = property on="PixelFormat" class="Ring (strict)"() -> ("RingText.Text"=w931:string)  [unwired: 2 in, 2 out]
                n463 = call "SetEnumFeatureSymbol.vi"("pEnumSymbol"=w931, "pFeatureName"=w932, "handle"=w934, "error in (no error)"=w935) -> ("error out"=w933:errorcluster)  [unwired: 6 in, 1 out]
                n464 = call "SetEnumFeatureSymbol.vi"("pEnumSymbol"=w931, "pFeatureName"=w932, "handle"=w930, "error in (no error)"=w933) -> ("error out"=w929:errorcluster)  [unwired: 6 in, 1 out]
              }
            }
          }
        }
      }
      event "PixelFormat 2": Value Change {
        n465 = event-data() -> ()  [unwired: 1 in, 6 out]
        n466 = local read "hIFDev 2"() -> (w937:i64)
        n467 = local read "hDev 2"() -> (w936:i64)
        n468 = Not Equal To 0?(x=w937) -> (x != 0?=w939:bool)
        n469 = Not Equal To 0?(x=w936) -> (x != 0?=w940:bool)
        n470 = And(x=w939, y=w940) -> (x .and. y?=w941:bool)
        n471 = case shown="True" w941 {
          tunnel: [errorcluster {FALSE, 0, "设备句柄为空"} w946] -> _
          tunnel: w937 -> [_ w943]
          tunnel: w936 -> [_ w945]
          tunnel: w938 -> [_ w944]
          frame False {
          }
          frame True {
            n472 = call "IsOpenInterface.vi"("interface handle"=w943, "error in (no error)"=w944) -> ("return type"=w952:i8, "error out"=w949:errorcluster)  [unwired: 8 in]
            n473 = Not Equal To 0?(x=w952) -> (x != 0?=w950:bool)
            n474 = call "IsDeviceOpen.vi"("dev handle"=w945, "error in (no error)"=w949) -> ("return type"=w953:i8, "error out"=w947:errorcluster)  [unwired: 8 in]
            n475 = Not Equal To 0?(x=w953) -> (x != 0?=w951:bool)
            n476 = And(x=w951, y=w950) -> (x .and. y?=w948:bool)
            n477 = case shown="True" w948 {
              tunnel: w947 -> [w954 w961]
              tunnel: [w954 w955] -> w946
              tunnel: w945 -> [_ w960]
              tunnel: w943 -> [_ w956]
              frame False {
              }
              frame True {
                w958 = "PixelFormat" ("pFeatureName")
                n478 = property on="PixelFormat 2" class="Ring (strict)"() -> ("RingText.Text"=w957:string)  [unwired: 2 in, 2 out]
                n479 = call "SetEnumFeatureSymbol.vi"("pEnumSymbol"=w957, "pFeatureName"=w958, "handle"=w960, "error in (no error)"=w961) -> ("error out"=w959:errorcluster)  [unwired: 6 in, 1 out]
                n480 = call "SetEnumFeatureSymbol.vi"("pEnumSymbol"=w957, "pFeatureName"=w958, "handle"=w956, "error in (no error)"=w959) -> ("error out"=w955:errorcluster)  [unwired: 6 in, 1 out]
              }
            }
          }
        }
      }
      event "TriggerSource": Value Change {
        n481 = event-data() -> ()  [unwired: 1 in, 6 out]
        n482 = local read "hIFDev 2"() -> (w964:i64)
        n483 = local read "hDev 2"() -> (w963:i64)
        n484 = local read "hIFDev"() -> (w972:i64)
        n485 = local read "hDev"() -> (w971:i64)
        n486 = Not Equal To 0?(x=w964) -> (x != 0?=w969:bool)
        n487 = Not Equal To 0?(x=w963) -> (x != 0?=w968:bool)
        n488 = Not Equal To 0?(x=w972) -> (x != 0?=w974:bool)
        n489 = Not Equal To 0?(x=w971) -> (x != 0?=w973:bool)
        n490 = And(x=w969, y=w968) -> (x .and. y?=w966:bool)
        n491 = And(x=w974, y=w973) -> (x .and. y?=w967:bool)
        n492 = And(x=w967, y=w966) -> (x .and. y?=w965:bool)
        n493 = case shown="True" w965 {
          tunnel: w972 -> [_ w991]
          tunnel: w971 -> [_ w986]
          tunnel: [errorcluster {"status"=FALSE, "code"=0, "source"="设备句柄为空"} ("error in") w985] -> w970
          tunnel: w962 -> [_ w989]
          tunnel: w964 -> [_ w979]
          tunnel: w963 -> [_ w976]
          tunnel: w962 -> [_ w978]
          frame False {
          }
          frame True {
            n494 = call "IsOpenInterface.vi"("interface handle"=w979, "error in (no error)"=w978) -> ("return type"=w982:i8, "error out"=w980:errorcluster)  [unwired: 8 in]
            n495 = call "IsOpenInterface.vi"("interface handle"=w991, "error in (no error)"=w989) -> ("return type"=w993:i8, "error out"=w988:errorcluster)  [unwired: 8 in]
            n496 = Not Equal To 0?(x=w982) -> (x != 0?=w984:bool)
            n497 = call "IsDeviceOpen.vi"("dev handle"=w976, "error in (no error)"=w980) -> ("return type"=w981:i8, "error out"=w977:errorcluster)  [unwired: 8 in]
            n498 = Not Equal To 0?(x=w993) -> (x != 0?=w995:bool)
            n499 = call "IsDeviceOpen.vi"("dev handle"=w986, "error in (no error)"=w988) -> ("return type"=w992:i8, "error out"=w987:errorcluster)  [unwired: 8 in]
            n500 = Not Equal To 0?(x=w981) -> (x != 0?=w983:bool)
            n501 = Not Equal To 0?(x=w992) -> (x != 0?=w994:bool)
            n502 = And(x=w983, y=w984) -> ()  [unwired: 1 out]
            n503 = And(x=w994, y=w995) -> (x .and. y?=w990:bool)
            n504 = case shown="True" w990 {
              tunnel: w987 -> [w996 w1027]
              tunnel: w986 -> [_ w1017]
              tunnel: [w996 w1014] -> w985
              tunnel: w977 -> [_ w998]
              tunnel: w976 -> [_ w997]
              frame False {
              }
              frame True {
                n505 = property on="TriggerSource" class="Ring (strict)"() -> ("RingText.Text"=w1025:string)  [unwired: 2 in, 2 out]
                n506 = property on="TriggerSource" class="Ring (strict)"() -> ("RingText.Text"=w1010:string)  [unwired: 2 in, 2 out]
                n507 = call "SetEnumFeatureSymbol.vi"("pEnumSymbol"=w1025, "pFeatureName"="TriggerSource", "handle"=w1017, "error in (no error)"=w1027) -> ("error out"=w1024:errorcluster)  [unwired: 6 in, 1 out]
                n508 = call "SetEnumFeatureSymbol.vi"("pEnumSymbol"=w1010, "pFeatureName"="TriggerSource", "handle"=w997, "error in (no error)"=w998) -> ("error out"=w1009:errorcluster)  [unwired: 6 in, 1 out]
                n509 = call "SetEnumFeatureSymbol.vi"("pEnumSymbol"="FrameStart", "pFeatureName"="TriggerSelector", "handle"=w1017, "error in (no error)"=w1024) -> ("error out"=w1021:errorcluster)  [unwired: 6 in, 1 out]
                n510 = call "SetEnumFeatureSymbol.vi"("pEnumSymbol"="FrameStart", "pFeatureName"="TriggerSelector", "handle"=w997, "error in (no error)"=w1009) -> ("error out"=w1006:errorcluster)  [unwired: 6 in, 1 out]
                n511 = call "SetEnumFeatureSymbol.vi"("pEnumSymbol"="On", "pFeatureName"="TriggerMode", "handle"=w1017, "error in (no error)"=w1021) -> ("return type"=w1012:i32, "error out"=w1020:errorcluster)  [unwired: 6 in]
                n512 = Equal To 0?(x=w1012) -> (x = 0?=w1013:bool)
                n513 = call "SetEnumFeatureSymbol.vi"("pEnumSymbol"="On", "pFeatureName"="TriggerMode", "handle"=w997, "error in (no error)"=w1006) -> ("return type"=w1000:i32, "error out"=w1005:errorcluster)  [unwired: 6 in]
                n514 = case shown="True" w1013 {
                  frame False {
                  }
                  frame True {
                    n515 = local write "TrigModeOn"(TRUE ("TrigModeOn")) -> ()
                  }
                }
                n516 = Equal To 0?(x=w1000) -> (x = 0?=w999:bool)
                n517 = case shown="True" w999 {
                  frame False {
                  }
                  frame True {
                    n518 = local write "TrigModeOn 2"(TRUE ("TrigModeOn 2")) -> ()
                  }
                }
                n519 = call "SetEnumFeatureSymbol.vi"("pEnumSymbol"="RisingEdge", "pFeatureName"="TriggerActivation", "handle"=w1017, "error in (no error)"=w1020) -> ("error out"=w1014:errorcluster)  [unwired: 6 in, 1 out]
                n520 = call "SetEnumFeatureSymbol.vi"("pEnumSymbol"="RisingEdge", "pFeatureName"="TriggerActivation", "handle"=w997, "error in (no error)"=w1005) -> ()  [unwired: 6 in, 2 out]
              }
            }
          }
        }
      }
      event "ExposureAuto": Value Change {
        n521 = event-data() -> ()  [unwired: 1 in, 6 out]
        n522 = local read "hIFDev"() -> (w1033:i64)
        n523 = local read "hDev"() -> (w1032:i64)
        n524 = Not Equal To 0?(x=w1033) -> (x != 0?=w1035:bool)
        n525 = Not Equal To 0?(x=w1032) -> (x != 0?=w1036:bool)
        n526 = And(x=w1035, y=w1036) -> (x .and. y?=w1034:bool)
        n527 = case shown="True" w1034 {
          tunnel: w1033 -> [_ w1042]
          tunnel: w1032 -> [_ w1038]
          tunnel: [errorcluster {"status"=FALSE, "code"=0, "source"="设备句柄为空"} ("error in") w1039] -> w1031
          tunnel: w1030 -> [_ w1043]
          frame False {
          }
          frame True {
            n528 = call "IsOpenInterface.vi"("interface handle"=w1042, "error in (no error)"=w1043) -> ("return type"=w1046:i8, "error out"=w1048:errorcluster)  [unwired: 8 in]
            n529 = Not Equal To 0?(x=w1046) -> (x != 0?=w1044:bool)
            n530 = call "IsDeviceOpen.vi"("dev handle"=w1038, "error in (no error)"=w1048) -> ("return type"=w1047:i8, "error out"=w1040:errorcluster)  [unwired: 8 in]
            n531 = Not Equal To 0?(x=w1047) -> (x != 0?=w1045:bool)
            n532 = And(x=w1045, y=w1044) -> (x .and. y?=w1041:bool)
            n533 = case shown="True" w1041 {
              tunnel: [w1049 w1053] -> w1039
              tunnel: w1040 -> [w1049 w1054]
              tunnel: w1038 -> [_ w1052]
              frame False {
              }
              frame True {
                n534 = property on="ExposureAuto" class="Ring (strict)"() -> ("RingText.Text"=w1050:string)  [unwired: 2 in, 2 out]
                n535 = call "SetEnumFeatureSymbol.vi"("pEnumSymbol"=w1050, "pFeatureName"="ExposureAuto", "handle"=w1052, "error in (no error)"=w1054) -> ("error out"=w1053:errorcluster)  [unwired: 6 in, 1 out]
              }
            }
          }
        }
      }
      event "ExposureAuto 2": Value Change {
        n536 = event-data() -> ()  [unwired: 1 in, 6 out]
        n537 = local read "hIFDev 2"() -> (w1057:i64)
        n538 = local read "hDev 2"() -> (w1056:i64)
        n539 = Not Equal To 0?(x=w1057) -> (x != 0?=w1059:bool)
        n540 = Not Equal To 0?(x=w1056) -> (x != 0?=w1060:bool)
        n541 = And(x=w1059, y=w1060) -> (x .and. y?=w1058:bool)
        n542 = case shown="True" w1058 {
          tunnel: w1057 -> [_ w1066]
          tunnel: w1056 -> [_ w1062]
          tunnel: [errorcluster {"status"=FALSE, "code"=0, "source"="设备句柄为空"} ("error in") w1063] -> _
          tunnel: w1055 -> [_ w1067]
          frame False {
          }
          frame True {
            n543 = call "IsOpenInterface.vi"("interface handle"=w1066, "error in (no error)"=w1067) -> ("return type"=w1070:i8, "error out"=w1072:errorcluster)  [unwired: 8 in]
            n544 = Not Equal To 0?(x=w1070) -> (x != 0?=w1068:bool)
            n545 = call "IsDeviceOpen.vi"("dev handle"=w1062, "error in (no error)"=w1072) -> ("return type"=w1071:i8, "error out"=w1064:errorcluster)  [unwired: 8 in]
            n546 = Not Equal To 0?(x=w1071) -> (x != 0?=w1069:bool)
            n547 = And(x=w1069, y=w1068) -> (x .and. y?=w1065:bool)
            n548 = case shown="True" w1065 {
              tunnel: [w1073 w1077] -> w1063
              tunnel: w1064 -> [w1073 w1078]
              tunnel: w1062 -> [_ w1076]
              frame False {
              }
              frame True {
                n549 = property on="ExposureAuto 2" class="Ring (strict)"() -> ("RingText.Text"=w1074:string)  [unwired: 2 in, 2 out]
                n550 = call "SetEnumFeatureSymbol.vi"("pEnumSymbol"=w1074, "pFeatureName"="ExposureAuto", "handle"=w1076, "error in (no error)"=w1078) -> ("error out"=w1077:errorcluster)  [unwired: 6 in, 1 out]
              }
            }
          }
        }
      }
    }
    n551 = local write "error out"(w651) -> ()
    n552 = local read "QuitFlag"() -> (w650:bool)
    n553 = Wait (ms)(milliseconds to wait=u32 10 ("等待时间（毫秒）")) -> ()  [unwired: 1 out]
  }
  n554 = while {
    tunnel: w1 -> [w1082]
    stop <- w1081 stop-if-true
    # "操作按钮值改变"
    n555 = event shown="[4] \"Play\": Value Change" {
      selector: _ -> [_ _ _ _ _ _ _ _ _ _]
      dyn-events: _ -> [_ _ _ _ _ _ _ _ _ _]
      timeout: _ -> [_ _ _ _ _ _ _ _ _ _]
      tunnel: [errorcluster {FALSE, 0, "Timeout"} w1088 w1110 w1211 w1266 w1368 w1404 w1438 w1454 w1462] -> w1079
      tunnel: w1082 -> [_ w1091 w1109 w1216 w1265 w1386 w1407 w1441 w1457 w1465]
      event Timeout {
        n556 = event-data() -> ()  [unwired: 1 in, 3 out]
      }
      event "Discovery": Value Change {
        n557 = event-data() -> ()  [unwired: 1 in, 6 out]
        n558 = property on="DeviceInterfaceType" class="Ring (strict)"(error in=w1091) -> (error out=w1094:errorcluster, "Value"=w1093:u16)  [unwired: 1 in, 1 out]
        n559 = case shown="3" w1093 {
          tunnel: [u32 1 u32 2 u32 4 u32 8] -> w1092
          frame 0, Default {
          }
          frame 1 {
          }
          frame 2 {
          }
          frame 3 {
          }
        }
        n560 = call "EnumInterface.vi"("nInterfaceType"=w1092, "error in"=w1094) -> ("nInterfaceNum"=w1085:u32, "interfaceKeyList"=→"interfaceKeyList":string[], "error out"=w1096:errorcluster)  [unwired: 7 in]
        "nInterfaceNum" <- w1085
        n561 = Not Equal To 0?(x=w1085) -> (x != 0?=w1087:bool)
        n562 = case shown="False" w1087 {
          frame False {
            n563 = One Button Dialog(message="未发现采集卡") -> ()  [unwired: 1 in, 1 out]
          }
          frame True {
            n564 = local write "HasInterface"(TRUE ("HasInterface")) -> ()
          }
        }
        n565 = call "EnumDevices.vi"("nDeviceType"=w1092, "error in"=w1096) -> ("nDeviceNum"=w1084:i32, "deviceKeyList"=w1090:string[], "error out"=w1097:errorcluster)  [unwired: 7 in]
        n566 = property on="DeviceList" class="Ring (strict)"(error in=w1097, "Strings []"=w1090) -> (error out=w1089:errorcluster)  [unwired: 1 in, 1 out]
        n567 = Not Equal To 0?(x=w1084) -> (x != 0?=w1086:bool)
        n568 = case shown="False" w1086 {
          frame False {
            n569 = One Button Dialog(message="未发现相机") -> ()  [unwired: 1 in, 1 out]
          }
          frame True {
            n570 = local write "HasDevices"(TRUE ("HasDevices")) -> ()
          }
        }
        n571 = property on="DeviceList 2" class="Ring (strict)"(error in=w1089, "Strings []"=w1090) -> (error out=w1088:errorcluster)  [unwired: 1 in, 1 out]
      }
      event "Open": Value Change {
        n572 = event-data() -> ()  [unwired: 1 in, 6 out]
        n573 = local read "DeviceOpened 2"() -> (w1107:bool)
        n574 = local read "DeviceOpened"() -> (w1108:bool)
        n575 = Not And(1:w1107, 2:w1108) -> (0:w1106:bool)
        n576 = case shown="True" w1106 {
          tunnel: [w1112 w1117] -> w1110
          tunnel: w1109 -> [w1112 w1113]
          frame False {
            n577 = One Button Dialog(message="相机已经打开，请勿重复操作") -> ()  [unwired: 1 in, 1 out]
          }
          frame True {
            n578 = local read "nInterfaceNum"() -> (w1118:u32)
            n579 = local read "interfaceKeyList"() -> (w1119:string[])
            n580 = while {
              tunnel: w1119 -> [w1200]
              tunnel: [w1197] -> w1116
              tunnel: w1118 -> [w1198]
              i -> [w1197]
              stop <- w1194 stop-if-true
              n581 = property on="DeviceList 2" class="Ring (strict)"() -> ("RingText.Text"=w1193:string)  [unwired: 2 in, 2 out]
              n582 = Index Array(array=w1200, index=w1197) -> (element=w1199:string)
              n583 = Search/Split String(string=w1193, search string/char (-)="[") -> (substring before match=w1191:string)  [unwired: 1 in, 2 out]
              n584 = Equal?(x=w1199, y=w1191) -> (x = y?=w1196:bool)
              n585 = Greater Or Equal?(x=w1197, y=w1198) -> (x >= y?=w1195:bool)
              n586 = Or(x=w1196, y=w1195) -> (x .or. y?=w1194:bool)
            }
            n587 = while {
              tunnel: w1119 -> [w1210]
              tunnel: [w1207] -> w1115
              tunnel: w1118 -> [w1208]
              i -> [w1207]
              stop <- w1204 stop-if-true
              n588 = property on="DeviceList" class="Ring (strict)"() -> ("RingText.Text"=w1203:string)  [unwired: 2 in, 2 out]
              n589 = Index Array(array=w1210, index=w1207) -> (element=w1209:string)
              n590 = Search/Split String(string=w1203, search string/char (-)="[") -> (substring before match=w1201:string)  [unwired: 1 in, 2 out]
              n591 = Equal?(x=w1209, y=w1201) -> (x = y?=w1206:bool)
              n592 = Greater Or Equal?(x=w1207, y=w1208) -> (x >= y?=w1205:bool)
              n593 = Or(x=w1206, y=w1205) -> (x .or. y?=w1204:bool)
            }
            n594 = Not Equal?(x=w1115, y=w1116) -> (x != y?=w1114:bool)
            n595 = case shown="True" w1114 {
              tunnel: w1115 -> [_ w1157]
              tunnel: w1116 -> [_ w1150]
              tunnel: w1113 -> [w1121 w1135]
              tunnel: [w1121 w1130] -> w1117
              tunnel: w1113 -> [_ w1122]
              frame False {
                n596 = One Button Dialog(message="选择的设备相同") -> ()  [unwired: 1 in, 1 out]
              }
              frame True {
                (unwired) T6."Enabled" ("Disabled")
                (unwired) T6."Enabled" ("Disabled")
                n597 = call "OpenInterface.vi"("nIndex"=w1157, "error in (no error)"=w1135) -> ("return type"=w1126:i32, "hIFDev"=→"hIFDev":i64, "error out"=w1176:errorcluster)  [unwired: 7 in]
                n598 = call "OpenInterface.vi"("nIndex"=w1150, "error in (no error)"=w1122) -> ("return type"=w1125:i32, "hIFDev"=→"hIFDev 2":i64, "error out"=w1149:errorcluster)  [unwired: 7 in]
                n599 = property on="DeviceList" class="Ring (strict)"() -> ("Value"=w1174:i64)  [unwired: 2 in, 2 out]
                n600 = property on="DeviceList 2" class="Ring (strict)"() -> ("Value"=w1155:i64)  [unwired: 2 in, 2 out]
                n601 = Equal To 0?(x=w1126) -> (x = 0?=w1171:bool)
                n602 = Equal To 0?(x=w1125) -> (x = 0?=w1152:bool)
                n603 = call "OpenDevice.vi"("pIdentifier"=w1174, "mode"=0, "error in (no error)"=w1176) -> ("return type"=w1124:i32, "hDev"=→"hDev":i64, "error out"=w1134:errorcluster)  [unwired: 6 in]
                n604 = Equal To 0?(x=w1124) -> (x = 0?=w1172:bool)
                n605 = call "OpenDevice.vi"("pIdentifier"=w1155, "mode"=0, "error in (no error)"=w1149) -> ("return type"=w1123:i32, "hDev"=→"hDev 2":i64, "error out"=w1133:errorcluster)  [unwired: 6 in]
                n606 = Equal To 0?(x=w1123) -> (x = 0?=w1153:bool)
                n607 = And(x=w1172, y=w1171) -> (x .and. y?=w1129:bool)
                n608 = And(x=w1153, y=w1152) -> (x .and. y?=w1151:bool)
                n609 = case shown="True" w1151 {
                  tunnel: w1123 -> [w1177 _]
                  frame False {
                    n610 = Number To Decimal String(number=w1177) -> (decimal integer string=w1178:string)  [unwired: 1 in]
                    n611 = Concatenate Strings("打开相机2失败" ("string"), w1178) -> (w1180:string)
                    n612 = One Button Dialog(message=w1180) -> ()  [unwired: 1 in, 1 out]
                  }
                  frame True {
                    n613 = local write "DeviceOpened 2"(TRUE ("DeviceOpened")) -> ()
                    n614 = local write "InterfaceOpened 2"(TRUE ("InterfaceOpened")) -> ()
                    n615 = local write "ResumeFlag 2"(TRUE ("ResumeFlag")) -> ()
                  }
                }
                n616 = case shown="True" w1129 {
                  tunnel: w1124 -> [w1184 _]
                  frame False {
                    n617 = Number To Decimal String(number=w1184) -> (decimal integer string=w1185:string)  [unwired: 1 in]
                    n618 = Concatenate Strings("打开相机1失败" ("string"), w1185) -> (w1187:string)
                    n619 = One Button Dialog(message=w1187) -> ()  [unwired: 1 in, 1 out]
                  }
                  frame True {
                    n620 = local write "DeviceOpened"(TRUE ("DeviceOpened")) -> ()
                    n621 = local write "InterfaceOpened"(TRUE ("InterfaceOpened")) -> ()
                    n622 = local write "ResumeFlag"(TRUE ("ResumeFlag")) -> ()
                  }
                }
                n623 = property on="DeviceScanType 2" class="Ring (strict)"(error in=w1133, "DisabledEnum"=T6."Enabled" ("Disabled")) -> (error out=w1138:errorcluster)  [unwired: 1 in, 1 out]
                n624 = property on="DeviceScanType" class="Ring (strict)"(error in=w1134, "DisabledEnum"=T6."Enabled" ("Disabled")) -> (error out=w1160:errorcluster)  [unwired: 1 in, 1 out]
                n625 = property on="GainRaw 2" class="DigNum (strict)"(error in=w1138, "DisabledEnum"=T6."Enabled" ("Disabled")) -> (error out=w1136:errorcluster)  [unwired: 1 in, 1 out]
                n626 = property on="GainRaw" class="DigNum (strict)"(error in=w1160, "DisabledEnum"=T6."Enabled" ("Disabled")) -> (error out=w1158:errorcluster)  [unwired: 1 in, 1 out]
                n627 = property on="Width 2" class="DigNum (strict)"(error in=w1136, "DisabledEnum"=T6."Enabled" ("Disabled")) -> (error out=w1144:errorcluster)  [unwired: 1 in, 1 out]
                n628 = property on="Width" class="DigNum (strict)"(error in=w1158, "DisabledEnum"=T6."Enabled" ("Disabled")) -> (error out=w1166:errorcluster)  [unwired: 1 in, 1 out]
                n629 = property on="Height 2" class="DigNum (strict)"(error in=w1144, "DisabledEnum"=T6."Enabled" ("Disabled")) -> (error out=w1139:errorcluster)  [unwired: 1 in, 1 out]
                n630 = property on="Height" class="DigNum (strict)"(error in=w1166, "DisabledEnum"=T6."Enabled" ("Disabled")) -> (error out=w1161:errorcluster)  [unwired: 1 in, 1 out]
                n631 = property on="ExposureTime 2" class="DigNum (strict)"(error in=w1139, "DisabledEnum"=T6."Enabled" ("Disabled")) -> (error out=w1145:errorcluster)  [unwired: 1 in, 1 out]
                n632 = property on="ExposureTime" class="DigNum (strict)"(error in=w1161, "DisabledEnum"=T6."Enabled" ("Disabled")) -> (error out=w1167:errorcluster)  [unwired: 1 in, 1 out]
                n633 = property on="PixelFormat" class="Ring (strict)"(error in=w1167, "DisabledEnum"=T6."Enabled" ("Disabled")) -> (error out=w1169:errorcluster)  [unwired: 1 in, 1 out]
                n634 = property on="PixelFormat 2" class="Ring (strict)"(error in=w1145, "DisabledEnum"=T6."Enabled" ("Disabled")) -> (error out=w1147:errorcluster)  [unwired: 1 in, 1 out]
                n635 = property on="ExposureAuto" class="Ring (strict)"(error in=w1169, "DisabledEnum"=T6."Enabled" ("Disabled")) -> (error out=w1132:errorcluster)  [unwired: 1 in, 1 out]
                n636 = property on="ExposureAuto 2" class="Ring (strict)"(error in=w1147, "DisabledEnum"=T6."Enabled" ("Disabled")) -> (error out=w1131:errorcluster)  [unwired: 1 in, 1 out]
                n637 = Merge Errors(w1132, w1131) -> (w1130:errorcluster)
              }
            }
          }
        }
      }
      event "Close": Value Change {
        (unwired) T6."Disabled and Grayed Out" ("Disabled")
        (unwired) T6."Disabled and Grayed Out" ("Disabled")
        n638 = event-data() -> ()  [unwired: 1 in, 6 out]
        n639 = local read "hDev 2"() -> (w1235:i64)
        n640 = local read "hDev"() -> (w1254:i64)
        n641 = call "CloseDevice.vi"("dev handle"=w1235, "error in (no error)"=w1216) -> ("return type"=w1234:i32, "error out"=w1230:errorcluster)  [unwired: 8 in]
        n642 = call "CloseDevice.vi"("dev handle"=w1254, "error in (no error)"=w1216) -> ("return type"=w1251:i32, "error out"=w1253:errorcluster)  [unwired: 8 in]
        n643 = local read "hIFDev 2"() -> (w1231:i64)
        n644 = local read "hIFDev"() -> (w1252:i64)
        n645 = call "CloseInterface.vi"("interface handle"=w1231, "error in (no error)"=w1230) -> ("return type"=w1232:i32, "error out"=w1215:errorcluster)  [unwired: 8 in]
        n646 = call "CloseInterface.vi"("interface handle"=w1252, "error in (no error)"=w1253) -> ("return type"=w1249:i32, "error out"=w1214:errorcluster)  [unwired: 8 in]
        n647 = Equal To 0?(x=w1234) -> (x = 0?=w1233:bool)
        n648 = Equal To 0?(x=w1251) -> (x = 0?=w1250:bool)
        n649 = case shown="True" w1250 {
          tunnel: w1249 -> [_ w1263]
          frame False {
          }
          frame True {
            n650 = Equal To 0?(x=w1263) -> (x = 0?=w1262:bool)
            n651 = local write "DeviceOpened"(FALSE ("DeviceOpened")) -> ()
            n652 = local write "ResumeFlag"(FALSE ("ResumeFlag")) -> ()
            n653 = case shown="True" w1262 {
              frame False {
              }
              frame True {
                n654 = local write "InterfaceOpened"(FALSE ("InterfaceOpened")) -> ()
              }
            }
          }
        }
        n655 = case shown="True" w1233 {
          tunnel: w1232 -> [_ w1258]
          frame False {
          }
          frame True {
            n656 = Equal To 0?(x=w1258) -> (x = 0?=w1257:bool)
            n657 = local write "DeviceOpened 2"(FALSE ("DeviceOpened")) -> ()
            n658 = local write "ResumeFlag 2"(FALSE ("ResumeFlag")) -> ()
            n659 = case shown="True" w1257 {
              frame False {
              }
              frame True {
                n660 = local write "InterfaceOpened 2"(FALSE ("InterfaceOpened")) -> ()
              }
            }
          }
        }
        n661 = property on="DeviceScanType 2" class="Ring (strict)"(error in=w1215, "DisabledEnum"=T6."Disabled and Grayed Out" ("Disabled")) -> (error out=w1219:errorcluster)  [unwired: 1 in, 1 out]
        n662 = property on="DeviceScanType" class="Ring (strict)"(error in=w1214, "DisabledEnum"=T6."Disabled and Grayed Out" ("Disabled")) -> (error out=w1238:errorcluster)  [unwired: 1 in, 1 out]
        n663 = property on="ExposureTime 2" class="DigNum (strict)"(error in=w1219, "DisabledEnum"=T6."Disabled and Grayed Out" ("Disabled")) -> (error out=w1217:errorcluster)  [unwired: 1 in, 1 out]
        n664 = property on="ExposureTime" class="DigNum (strict)"(error in=w1238, "DisabledEnum"=T6."Disabled and Grayed Out" ("Disabled")) -> (error out=w1236:errorcluster)  [unwired: 1 in, 1 out]
        n665 = property on="PixelFormat 2" class="Ring (strict)"(error in=w1217, "DisabledEnum"=T6."Disabled and Grayed Out" ("Disabled")) -> (error out=w1225:errorcluster)  [unwired: 1 in, 1 out]
        n666 = property on="PixelFormat" class="Ring (strict)"(error in=w1236, "DisabledEnum"=T6."Disabled and Grayed Out" ("Disabled")) -> (error out=w1244:errorcluster)  [unwired: 1 in, 1 out]
        n667 = property on="Width 2" class="DigNum (strict)"(error in=w1225, "DisabledEnum"=T6."Disabled and Grayed Out" ("Disabled")) -> (error out=w1220:errorcluster)  [unwired: 1 in, 1 out]
        n668 = property on="Width" class="DigNum (strict)"(error in=w1244, "DisabledEnum"=T6."Disabled and Grayed Out" ("Disabled")) -> (error out=w1239:errorcluster)  [unwired: 1 in, 1 out]
        n669 = property on="Height 2" class="DigNum (strict)"(error in=w1220, "DisabledEnum"=T6."Disabled and Grayed Out" ("Disabled")) -> (error out=w1226:errorcluster)  [unwired: 1 in, 1 out]
        n670 = property on="Height" class="DigNum (strict)"(error in=w1239, "DisabledEnum"=T6."Disabled and Grayed Out" ("Disabled")) -> (error out=w1245:errorcluster)  [unwired: 1 in, 1 out]
        n671 = property on="GainRaw 2" class="DigNum (strict)"(error in=w1226, "DisabledEnum"=T6."Disabled and Grayed Out" ("Disabled")) -> (error out=w1228:errorcluster)  [unwired: 1 in, 1 out]
        n672 = property on="GainRaw" class="DigNum (strict)"(error in=w1245, "DisabledEnum"=T6."Disabled and Grayed Out" ("Disabled")) -> (error out=w1247:errorcluster)  [unwired: 1 in, 1 out]
        n673 = property on="ExposureAuto 2" class="Ring (strict)"(error in=w1228, "DisabledEnum"=T6."Disabled and Grayed Out" ("Disabled")) -> (error out=w1212:errorcluster)  [unwired: 1 in, 1 out]
        n674 = property on="ExposureAuto" class="Ring (strict)"(error in=w1247, "DisabledEnum"=T6."Disabled and Grayed Out" ("Disabled")) -> (error out=w1213:errorcluster)  [unwired: 1 in, 1 out]
        n675 = Merge Errors(w1213, w1212) -> (w1211:errorcluster)
      }
      event "Play": Value Change {
        n676 = event-data() -> ()  [unwired: 1 in, 6 out]
        n677 = local read "hIFDev 2"() -> (w1275:i64)
        n678 = local read "hIFDev"() -> (w1277:i64)
        n679 = local read "hDev 2"() -> (w1274:i64)
        n680 = local read "hDev"() -> (w1276:i64)
        n681 = Not Equal To 0?(x=w1277) -> (x != 0?=w1278:bool)
        n682 = Not Equal To 0?(x=w1276) -> (x != 0?=w1279:bool)
        n683 = Not Equal To 0?(x=w1275) -> (x != 0?=w1273:bool)
        n684 = Not Equal To 0?(x=w1274) -> (x != 0?=w1272:bool)
        n685 = And(x=w1278, y=w1279) -> (x .and. y?=w1271:bool)
        n686 = And(x=w1273, y=w1272) -> (x .and. y?=w1270:bool)
        n687 = And(x=w1271, y=w1270) -> (x .and. y?=w1269:bool)
        n688 = case shown="True" w1269 {
          tunnel: w1277 -> [_ w1327]
          tunnel: w1276 -> [_ w1329]
          tunnel: [errorcluster {"status"=FALSE, "code"=0, "source"="未打开相机"} ("error out") w1326] -> w1268
          tunnel: w1265 -> [_ w1325]
          frame False {
          }
          frame True {
            n689 = call "IsOpenInterface.vi"("interface handle"=w1327, "error in (no error)"=w1325) -> ("return type"=w1333:i8, "error out"=w1324:errorcluster)  [unwired: 8 in]
            n690 = Not Equal To 0?(x=w1333) -> (x != 0?=w1332:bool)
            n691 = call "IsDeviceOpen.vi"("dev handle"=w1329, "error in (no error)"=w1324) -> ("return type"=w1330:i8, "error out"=w1323:errorcluster)  [unwired: 8 in]
            n692 = Not Equal To 0?(x=w1330) -> (x != 0?=w1331:bool)
            n693 = And(x=w1332, y=w1331) -> (x .and. y?=w1328:bool)
            n694 = case shown="True" w1328 {
              tunnel: w1327 -> [_ w1338]
              tunnel: [errorcluster {"status"=FALSE, "code"=0, "source"="未打开相机"} ("error out") w1340] -> w1326
              tunnel: w1323 -> [_ w1335]
              frame False {
              }
              frame True {
                n695 = call "IsGrabbing.vi"("interface handle"=w1338, "error in (no error)"=w1335) -> ("return type"=w1336:i8, "error out"=w1339:errorcluster)  [unwired: 8 in]
                n696 = Equal To 0?(x=w1336) -> (x = 0?=w1337:bool)
                n697 = case shown="True" w1337 {
                  tunnel: [w1341 w1348] -> w1340
                  tunnel: w1339 -> [w1341 w1345]
                  tunnel: w1338 -> [_ w1344]
                  frame False {
                  }
                  frame True {
                    n698 = call "SetBufferCount.vi"("nSize"=u32 2, "interface handle"=w1344, "error in (no error)"=w1345) -> ("error out"=w1347:errorcluster)  [unwired: 7 in, 1 out]
                    n699 = call "StartGrabbing.vi"("interface handle"=w1344, "error in (no error)"=w1347) -> ("return type"=w1343:i32, "error out"=w1351:errorcluster)  [unwired: 8 in]
                    n700 = Equal To 0?(x=w1343) -> (x = 0?=w1342:bool)
                    n701 = case shown="True" w1342 {
                      frame False {
                      }
                      frame True {
                        n702 = local write "IsGrabbing"(TRUE ("IsGrabbing")) -> ()
                      }
                    }
                    n703 = property on="ExposureAuto" class="Ring (strict)"(error in=w1351, "DisabledEnum"=T6."Enabled" ("Disabled")) -> (error out=w1350:errorcluster)  [unwired: 1 in, 1 out]
                    n704 = property on="DeviceScanType" class="Ring (strict)"(error in=w1350, "DisabledEnum"=T6."Enabled" ("Disabled")) -> (error out=w1358:errorcluster)  [unwired: 1 in, 1 out]
                    n705 = property on="ExposureTime" class="DigNum (strict)"(error in=w1358, "DisabledEnum"=T6."Enabled" ("Disabled")) -> (error out=w1359:errorcluster)  [unwired: 1 in, 1 out]
                    n706 = property on="GainRaw" class="DigNum (strict)"(error in=w1359, "DisabledEnum"=T6."Enabled" ("Disabled")) -> (error out=w1360:errorcluster)  [unwired: 1 in, 1 out]
                    n707 = property on="Width" class="DigNum (strict)"(error in=w1360, "DisabledEnum"=T6."Disabled and Grayed Out" ("Disabled")) -> (error out=w1361:errorcluster)  [unwired: 1 in, 1 out]
                    n708 = property on="Height" class="DigNum (strict)"(error in=w1361, "DisabledEnum"=T6."Disabled and Grayed Out" ("Disabled")) -> (error out=w1362:errorcluster)  [unwired: 1 in, 1 out]
                    n709 = property on="PixelFormat" class="Ring (strict)"(error in=w1362, "DisabledEnum"=T6."Disabled and Grayed Out" ("Disabled")) -> (error out=w1348:errorcluster)  [unwired: 1 in, 1 out]
                  }
                }
              }
            }
          }
        }
        n710 = case shown="True" w1269 {
          tunnel: [errorcluster {"status"=FALSE, "code"=0, "source"="未打开相机"} ("error out") w1286] -> w1267
          tunnel: w1275 -> [_ w1285]
          tunnel: w1274 -> [_ w1284]
          tunnel: w1265 -> [_ w1283]
          frame False {
          }
          frame True {
            n711 = call "IsOpenInterface.vi"("interface handle"=w1285, "error in (no error)"=w1283) -> ("return type"=w1291:i8, "error out"=w1282:errorcluster)  [unwired: 8 in]
            n712 = Not Equal To 0?(x=w1291) -> (x != 0?=w1290:bool)
            n713 = call "IsDeviceOpen.vi"("dev handle"=w1284, "error in (no error)"=w1282) -> ("return type"=w1288:i8, "error out"=w1281:errorcluster)  [unwired: 8 in]
            n714 = Not Equal To 0?(x=w1288) -> (x != 0?=w1289:bool)
            n715 = And(x=w1290, y=w1289) -> (x .and. y?=w1287:bool)
            n716 = case shown="True" w1287 {
              tunnel: w1285 -> [_ w1296]
              tunnel: [errorcluster {"status"=FALSE, "code"=0, "source"="未打开相机"} ("error out") w1298] -> w1286
              tunnel: w1281 -> [_ w1293]
              frame False {
              }
              frame True {
                n717 = call "IsGrabbing.vi"("interface handle"=w1296, "error in (no error)"=w1293) -> ("return type"=w1294:i8, "error out"=w1297:errorcluster)  [unwired: 8 in]
                n718 = Equal To 0?(x=w1294) -> (x = 0?=w1295:bool)
                n719 = case shown="True" w1295 {
                  tunnel: [w1299 w1306] -> w1298
                  tunnel: w1297 -> [w1299 w1303]
                  tunnel: w1296 -> [_ w1302]
                  frame False {
                  }
                  frame True {
                    n720 = call "SetBufferCount.vi"("nSize"=u32 2, "interface handle"=w1302, "error in (no error)"=w1303) -> ("error out"=w1305:errorcluster)  [unwired: 7 in, 1 out]
                    n721 = call "StartGrabbing.vi"("interface handle"=w1302, "error in (no error)"=w1305) -> ("return type"=w1300:i32, "error out"=w1309:errorcluster)  [unwired: 8 in]
                    n722 = Equal To 0?(x=w1300) -> (x = 0?=w1301:bool)
                    n723 = case shown="True" w1301 {
                      frame False {
                      }
                      frame True {
                        n724 = local write "IsGrabbing 2"(TRUE ("IsGrabbing 2")) -> ()
                      }
                    }
                    n725 = property on="ExposureAuto 2" class="Ring (strict)"(error in=w1309, "DisabledEnum"=T6."Enabled" ("Disabled")) -> (error out=w1308:errorcluster)  [unwired: 1 in, 1 out]
                    n726 = property on="DeviceScanType 2" class="Ring (strict)"(error in=w1308, "DisabledEnum"=T6."Enabled" ("Disabled")) -> (error out=w1316:errorcluster)  [unwired: 1 in, 1 out]
                    n727 = property on="ExposureTime 2" class="DigNum (strict)"(error in=w1316, "DisabledEnum"=T6."Enabled" ("Disabled")) -> (error out=w1317:errorcluster)  [unwired: 1 in, 1 out]
                    n728 = property on="GainRaw 2" class="DigNum (strict)"(error in=w1317, "DisabledEnum"=T6."Enabled" ("Disabled")) -> (error out=w1318:errorcluster)  [unwired: 1 in, 1 out]
                    n729 = property on="Width 2" class="DigNum (strict)"(error in=w1318, "DisabledEnum"=T6."Disabled and Grayed Out" ("Disabled")) -> (error out=w1319:errorcluster)  [unwired: 1 in, 1 out]
                    n730 = property on="Height 2" class="DigNum (strict)"(error in=w1319, "DisabledEnum"=T6."Disabled and Grayed Out" ("Disabled")) -> (error out=w1320:errorcluster)  [unwired: 1 in, 1 out]
                    n731 = property on="PixelFormat 2" class="Ring (strict)"(error in=w1320, "DisabledEnum"=T6."Disabled and Grayed Out" ("Disabled")) -> (error out=w1306:errorcluster)  [unwired: 1 in, 1 out]
                  }
                }
              }
            }
          }
        }
        n732 = Merge Errors(w1268, w1267) -> (w1266:errorcluster)
      }
      event "Stop": Value Change {
        n733 = event-data() -> ()  [unwired: 1 in, 6 out]
        n734 = local read "hIFDev 2"() -> (w1387:i64)
        n735 = local read "hIFDev"() -> (w1401:i64)
        n736 = call "StopGrabbing.vi"("interface handle"=w1387, "error in (no error)"=w1386) -> ("return type"=w1364:i32, "error out"=w1371:errorcluster)  [unwired: 8 in]
        n737 = call "StopGrabbing.vi"("interface handle"=w1401, "error in (no error)"=w1386) -> ("return type"=w1366:i32, "error out"=w1385:errorcluster)  [unwired: 8 in]
        n738 = Equal To 0?(x=w1364) -> (x = 0?=w1365:bool)
        n739 = Equal To 0?(x=w1366) -> (x = 0?=w1367:bool)
        n740 = case shown="True" w1365 {
          frame False {
          }
          frame True {
            n741 = local write "IsGrabbing 2"(FALSE ("IsGrabbing 2")) -> ()
          }
        }
        n742 = case shown="True" w1367 {
          frame False {
          }
          frame True {
            n743 = local write "IsGrabbing"(FALSE ("IsGrabbing")) -> ()
          }
        }
        n744 = property on="DeviceScanType 2" class="Ring (strict)"(error in=w1371, "DisabledEnum"=T6."Enabled" ("Disabled")) -> (error out=w1378:errorcluster)  [unwired: 1 in, 1 out]
        n745 = property on="DeviceScanType" class="Ring (strict)"(error in=w1385, "DisabledEnum"=T6."Enabled" ("Disabled")) -> (error out=w1394:errorcluster)  [unwired: 1 in, 1 out]
        n746 = property on="ExposureTime 2" class="DigNum (strict)"(error in=w1378, "DisabledEnum"=T6."Enabled" ("Disabled")) -> (error out=w1377:errorcluster)  [unwired: 1 in, 1 out]
        n747 = property on="ExposureTime" class="DigNum (strict)"(error in=w1394, "DisabledEnum"=T6."Enabled" ("Disabled")) -> (error out=w1393:errorcluster)  [unwired: 1 in, 1 out]
        n748 = property on="GainRaw 2" class="DigNum (strict)"(error in=w1377, "DisabledEnum"=T6."Enabled" ("Disabled")) -> (error out=w1376:errorcluster)  [unwired: 1 in, 1 out]
        n749 = property on="GainRaw" class="DigNum (strict)"(error in=w1393, "DisabledEnum"=T6."Enabled" ("Disabled")) -> (error out=w1392:errorcluster)  [unwired: 1 in, 1 out]
        n750 = property on="Width 2" class="DigNum (strict)"(error in=w1376, "DisabledEnum"=T6."Enabled" ("Disabled")) -> (error out=w1375:errorcluster)  [unwired: 1 in, 1 out]
        n751 = property on="Width" class="DigNum (strict)"(error in=w1392, "DisabledEnum"=T6."Enabled" ("Disabled")) -> (error out=w1391:errorcluster)  [unwired: 1 in, 1 out]
        n752 = property on="Height 2" class="DigNum (strict)"(error in=w1375, "DisabledEnum"=T6."Enabled" ("Disabled")) -> (error out=w1374:errorcluster)  [unwired: 1 in, 1 out]
        n753 = property on="Height" class="DigNum (strict)"(error in=w1391, "DisabledEnum"=T6."Enabled" ("Disabled")) -> (error out=w1390:errorcluster)  [unwired: 1 in, 1 out]
        n754 = property on="PixelFormat 2" class="Ring (strict)"(error in=w1374, "DisabledEnum"=T6."Enabled" ("Disabled")) -> (error out=w1373:errorcluster)  [unwired: 1 in, 1 out]
        n755 = property on="PixelFormat" class="Ring (strict)"(error in=w1390, "DisabledEnum"=T6."Enabled" ("Disabled")) -> (error out=w1389:errorcluster)  [unwired: 1 in, 1 out]
        n756 = property on="ExposureAuto 2" class="Ring (strict)"(error in=w1373, "DisabledEnum"=T6."Enabled" ("Disabled")) -> (error out=w1370:errorcluster)  [unwired: 1 in, 1 out]
        n757 = property on="ExposureAuto" class="Ring (strict)"(error in=w1389, "DisabledEnum"=T6."Enabled" ("Disabled")) -> (error out=w1369:errorcluster)  [unwired: 1 in, 1 out]
        n758 = Merge Errors(w1369, w1370) -> (w1368:errorcluster)
      }
      event "OpenTrig": Value Change {
        n759 = event-data() -> ()  [unwired: 1 in, 6 out]
        n760 = local read "hDev 2"() -> (w1408:i64)
        n761 = local read "hDev"() -> (w1424:i64)
        n762 = call "SetEnumFeatureSymbol.vi"("pEnumSymbol"="Software", "pFeatureName"="TriggerSource", "handle"=w1408, "error in (no error)"=w1407) -> ("error out"=w1411:errorcluster)  [unwired: 6 in, 1 out]
        n763 = call "SetEnumFeatureSymbol.vi"("pEnumSymbol"="Software", "pFeatureName"="TriggerSource", "handle"=w1424, "error in (no error)"=w1407) -> ("error out"=w1433:errorcluster)  [unwired: 6 in, 1 out]
        n764 = call "SetDoubleFeatureValue.vi"("doubleValue"=0.0, "pFeatureName"="LineDebouncerTime", "handle"=w1408, "error in (no error)"=w1411) -> ("error out"=w1414:errorcluster)  [unwired: 7 in]
        n765 = call "SetDoubleFeatureValue.vi"("doubleValue"=0.0, "pFeatureName"="LineDebouncerTime", "handle"=w1424, "error in (no error)"=w1433) -> ("error out"=w1430:errorcluster)  [unwired: 7 in]
        n766 = call "SetEnumFeatureSymbol.vi"("pEnumSymbol"="CC1", "pFeatureName"="LineSelector", "handle"=w1408, "error in (no error)"=w1414) -> ("error out"=w1417:errorcluster)  [unwired: 6 in, 1 out]
        n767 = call "SetEnumFeatureSymbol.vi"("pEnumSymbol"="CC1", "pFeatureName"="LineSelector", "handle"=w1424, "error in (no error)"=w1430) -> ("error out"=w1427:errorcluster)  [unwired: 6 in, 1 out]
        n768 = call "SetEnumFeatureSymbol.vi"("pEnumSymbol"="On", "pFeatureName"="TriggerMode", "handle"=w1408, "error in (no error)"=w1417) -> ("return type"=w1420:i32, "error out"=w1405:errorcluster)  [unwired: 6 in]
        n769 = call "SetEnumFeatureSymbol.vi"("pEnumSymbol"="On", "pFeatureName"="TriggerMode", "handle"=w1424, "error in (no error)"=w1427) -> ("return type"=w1423:i32, "error out"=w1406:errorcluster)  [unwired: 6 in]
        n770 = Equal To 0?(x=w1420) -> (x = 0?=w1421:bool)
        n771 = Equal To 0?(x=w1423) -> (x = 0?=w1422:bool)
        n772 = case shown="True" w1421 {
          frame False {
          }
          frame True {
            n773 = local write "TrigModeOn 2"(TRUE ("TrigModeOn")) -> ()
          }
        }
        n774 = case shown="True" w1422 {
          frame False {
          }
          frame True {
            n775 = local write "TrigModeOn"(TRUE ("TrigModeOn")) -> ()
          }
        }
        n776 = Merge Errors(w1406, w1405) -> (w1404:errorcluster)
      }
      event "CloseTrig": Value Change {
        n777 = event-data() -> ()  [unwired: 1 in, 6 out]
        n778 = local read "hDev 2"() -> (w1442:i64)
        n779 = local read "hDev"() -> (w1447:i64)
        n780 = call "SetEnumFeatureSymbol.vi"("pEnumSymbol"="Off", "pFeatureName"="TriggerMode", "handle"=w1442, "error in (no error)"=w1441) -> ("return type"=w1444:i32, "error out"=w1439:errorcluster)  [unwired: 6 in]
        n781 = call "SetEnumFeatureSymbol.vi"("pEnumSymbol"="Off", "pFeatureName"="TriggerMode", "handle"=w1447, "error in (no error)"=w1441) -> ("return type"=w1449:i32, "error out"=w1440:errorcluster)  [unwired: 6 in]
        n782 = Equal To 0?(x=w1444) -> (x = 0?=w1443:bool)
        n783 = Equal To 0?(x=w1449) -> (x = 0?=w1448:bool)
        n784 = case shown="True" w1443 {
          frame False {
          }
          frame True {
            n785 = local write "TrigModeOn 2"(FALSE ("TrigModeOn")) -> ()
          }
        }
        n786 = case shown="True" w1448 {
          frame False {
          }
          frame True {
            n787 = local write "TrigModeOn"(FALSE ("TrigModeOn")) -> ()
          }
        }
        n788 = Merge Errors(w1440, w1439) -> (w1438:errorcluster)
      }
      event "ExecuteSoftTrig": Value Change {
        n789 = event-data() -> ()  [unwired: 1 in, 6 out]
        n790 = local read "hDev 2"() -> (w1458:i64)
        n791 = local read "hDev"() -> (w1461:i64)
        n792 = call "ExecuteCommandFeature.vi"("pFeatureName"="TriggerSoftware", "handle"=w1461, "error in (no error)"=w1457) -> ("error out"=w1456:errorcluster)  [unwired: 7 in, 1 out]
        n793 = call "ExecuteCommandFeature.vi"("pFeatureName"="TriggerSoftware", "handle"=w1458, "error in (no error)"=w1457) -> ("error out"=w1455:errorcluster)  [unwired: 7 in, 1 out]
        n794 = Merge Errors(w1456, w1455) -> (w1454:errorcluster)
      }
      event "Quit": Value Change {
        n795 = event-data() -> ()  [unwired: 1 in, 6 out]
        n796 = flat-sequence {
          tunnel: w1465 -> [w1468]
          tunnel: [w1468] -> w1466
          tunnel: w1466 -> [w1479]
          tunnel: [w1475] -> w1463
          frame #0 {
            n797 = local write "SavePic"(FALSE ("SavePic")) -> ()
            n798 = Wait (ms)(milliseconds to wait=u32 500 ("等待时间（毫秒）")) -> ()  [unwired: 1 out]
          }
          frame #1 {
            (unwired) T6."Disabled and Grayed Out" ("Disabled")
            n799 = local read "hDev 2"() -> (w1484:i64)
            n800 = local read "hIFDev 2"() -> (w1483:i64)
            n801 = call "SetEnumFeatureSymbol.vi"("pEnumSymbol"="Off", "pFeatureName"="TriggerMode", "handle"=w1484, "error in (no error)"=w1479) -> ("return type"=w1499:i32, "error out"=w1500:errorcluster)  [unwired: 6 in]
            n802 = Equal To 0?(x=w1499) -> (x = 0?=w1498:bool)
            n803 = case shown="True" w1498 {
              frame False {
              }
              frame True {
                n804 = local write "TrigModeOn 2"(FALSE ("TrigModeOn 2")) -> ()
              }
            }
            n805 = call "StopGrabbing.vi"("interface handle"=w1483, "error in (no error)"=w1500) -> ("return type"=w1472:i32, "error out"=w1478:errorcluster)  [unwired: 8 in]
            n806 = Equal To 0?(x=w1472) -> (x = 0?=w1471:bool)
            n807 = case shown="True" w1471 {
              frame False {
              }
              frame True {
                n808 = local write "IsGrabbing 2"(FALSE ("IsGrabbing 2")) -> ()
              }
            }
            n809 = property on="ExposureAuto 2" class="Ring (strict)"(error in=w1478, "DisabledEnum"=T6."Disabled and Grayed Out" ("Disabled")) -> (error out=w1496:errorcluster)  [unwired: 1 in, 1 out]
            n810 = property on="DeviceScanType 2" class="Ring (strict)"(error in=w1496, "DisabledEnum"=T6."Disabled and Grayed Out" ("Disabled")) -> (error out=w1487:errorcluster)  [unwired: 1 in, 1 out]
            n811 = property on="PixelFormat 2" class="Ring (strict)"(error in=w1487, "DisabledEnum"=T6."Disabled and Grayed Out" ("Disabled")) -> (error out=w1485:errorcluster)  [unwired: 1 in, 1 out]
            n812 = property on="Height 2" class="DigNum (strict)"(error in=w1485, "DisabledEnum"=T6."Disabled and Grayed Out" ("Disabled")) -> (error out=w1493:errorcluster)  [unwired: 1 in, 1 out]
            n813 = property on="Width 2" class="DigNum (strict)"(error in=w1493, "DisabledEnum"=T6."Disabled and Grayed Out" ("Disabled")) -> (error out=w1488:errorcluster)  [unwired: 1 in, 1 out]
            n814 = property on="ExposureTime 2" class="DigNum (strict)"(error in=w1488, "DisabledEnum"=T6."Disabled and Grayed Out" ("Disabled")) -> (error out=w1494:errorcluster)  [unwired: 1 in, 1 out]
            n815 = property on="GainRaw 2" class="DigNum (strict)"(error in=w1494, "DisabledEnum"=T6."Disabled and Grayed Out" ("Disabled")) -> (error out=w1477:errorcluster)  [unwired: 1 in, 1 out]
            n816 = call "CloseDevice.vi"("dev handle"=w1484, "error in (no error)"=w1477) -> ("return type"=w1481:i32, "error out"=w1476:errorcluster)  [unwired: 8 in]
            n817 = Equal To 0?(x=w1481) -> (x = 0?=w1482:bool)
            n818 = call "CloseInterface.vi"("interface handle"=w1483, "error in (no error)"=w1476) -> ("return type"=w1480:i32, "error out"=w1475:errorcluster)  [unwired: 8 in]
            n819 = case shown="True" w1482 {
              tunnel: w1480 -> [_ w1505]
              frame False {
              }
              frame True {
                n820 = local write "DeviceOpened 2"(FALSE ("DeviceOpened 2")) -> ()
                n821 = local write "ResumeFlag 2"(FALSE ("ResumeFlag 2")) -> ()
                n822 = Equal To 0?(x=w1505) -> (x = 0?=w1504:bool)
                n823 = case shown="True" w1504 {
                  frame False {
                  }
                  frame True {
                    n824 = local write "InterfaceOpened 2"(FALSE ("InterfaceOpened 2")) -> ()
                  }
                }
              }
            }
            n825 = local write "QuitFlag"(FALSE ("QuitFlag")) -> ()
            n826 = property on="DeviceList 2" class="Ring (strict)"("Strings []"=string[] []) -> ()  [unwired: 2 in, 2 out]
          }
        }
        n827 = flat-sequence {
          tunnel: w1465 -> [w1510]
          tunnel: [w1510] -> w1467
          tunnel: w1467 -> [w1516]
          tunnel: [w1515] -> w1464
          frame #0 {
            n828 = local write "SavePic"(FALSE ("SavePic")) -> ()
            n829 = Wait (ms)(milliseconds to wait=u32 500 ("等待时间（毫秒）")) -> ()  [unwired: 1 out]
          }
          frame #1 {
            (unwired) T6."Disabled and Grayed Out" ("Disabled")
            n830 = local read "hDev"() -> (w1529:i64)
            n831 = call "SetEnumFeatureSymbol.vi"("pEnumSymbol"="Off", "pFeatureName"="TriggerMode", "handle"=w1529, "error in (no error)"=w1516) -> ("return type"=w1544:i32, "error out"=w1542:errorcluster)  [unwired: 6 in]
            n832 = local read "hIFDev"() -> (w1528:i64)
            n833 = Equal To 0?(x=w1544) -> (x = 0?=w1543:bool)
            n834 = case shown="True" w1543 {
              frame False {
              }
              frame True {
                n835 = local write "TrigModeOn"(FALSE ("TrigModeOn")) -> ()
              }
            }
            n836 = call "StopGrabbing.vi"("interface handle"=w1528, "error in (no error)"=w1542) -> ("return type"=w1513:i32, "error out"=w1520:errorcluster)  [unwired: 8 in]
            n837 = Equal To 0?(x=w1513) -> (x = 0?=w1514:bool)
            n838 = case shown="True" w1514 {
              frame False {
              }
              frame True {
                n839 = local write "IsGrabbing"(FALSE ("IsGrabbing")) -> ()
              }
            }
            n840 = property on="ExposureAuto" class="Ring (strict)"(error in=w1520, "DisabledEnum"=T6."Disabled and Grayed Out" ("Disabled")) -> (error out=w1519:errorcluster)  [unwired: 1 in, 1 out]
            n841 = property on="DeviceScanType" class="Ring (strict)"(error in=w1519, "DisabledEnum"=T6."Disabled and Grayed Out" ("Disabled")) -> (error out=w1539:errorcluster)  [unwired: 1 in, 1 out]
            n842 = property on="PixelFormat" class="Ring (strict)"(error in=w1539, "DisabledEnum"=T6."Disabled and Grayed Out" ("Disabled")) -> (error out=w1541:errorcluster)  [unwired: 1 in, 1 out]
            n843 = property on="Height" class="DigNum (strict)"(error in=w1541, "DisabledEnum"=T6."Disabled and Grayed Out" ("Disabled")) -> (error out=w1533:errorcluster)  [unwired: 1 in, 1 out]
            n844 = property on="Width" class="DigNum (strict)"(error in=w1533, "DisabledEnum"=T6."Disabled and Grayed Out" ("Disabled")) -> (error out=w1538:errorcluster)  [unwired: 1 in, 1 out]
            n845 = property on="ExposureTime" class="DigNum (strict)"(error in=w1538, "DisabledEnum"=T6."Disabled and Grayed Out" ("Disabled")) -> (error out=w1532:errorcluster)  [unwired: 1 in, 1 out]
            n846 = property on="GainRaw" class="DigNum (strict)"(error in=w1532, "DisabledEnum"=T6."Disabled and Grayed Out" ("Disabled")) -> (error out=w1530:errorcluster)  [unwired: 1 in, 1 out]
            n847 = call "CloseDevice.vi"("dev handle"=w1529, "error in (no error)"=w1530) -> ("return type"=w1525:i32, "error out"=w1527:errorcluster)  [unwired: 8 in]
            n848 = Equal To 0?(x=w1525) -> (x = 0?=w1526:bool)
            n849 = call "CloseInterface.vi"("interface handle"=w1528, "error in (no error)"=w1527) -> ("return type"=w1524:i32, "error out"=w1515:errorcluster)  [unwired: 8 in]
            n850 = case shown="True" w1526 {
              tunnel: w1524 -> [_ w1550]
              frame False {
              }
              frame True {
                n851 = local write "DeviceOpened"(FALSE ("DeviceOpened")) -> ()
                n852 = local write "ResumeFlag"(FALSE ("ResumeFlag")) -> ()
                n853 = Equal To 0?(x=w1550) -> (x = 0?=w1549:bool)
                n854 = case shown="True" w1549 {
                  frame False {
                  }
                  frame True {
                    n855 = local write "InterfaceOpened"(FALSE ("InterfaceOpened")) -> ()
                  }
                }
              }
            }
            n856 = local write "HasDevices"(FALSE ("HasDevices")) -> ()
            n857 = local write "HasInterface"(FALSE ("HasInterface")) -> ()
            n858 = local write "QuitFlag"(FALSE ("QuitFlag")) -> ()
            n859 = property on="DeviceList" class="Ring (strict)"("Strings []"=string[] []) -> ()  [unwired: 2 in, 2 out]
          }
        }
        n860 = Merge Errors(w1464, w1463) -> (w1462:errorcluster)
      }
    }
    n861 = local read "QuitFlag"() -> (w1081:bool)
    n862 = local write "error out"(w1079) -> ()
    n863 = Wait (ms)(milliseconds to wait=u32 10 ("等待时间（毫秒）")) -> ()  [unwired: 1 out]
  }
